vi "4Pi Capture Manager.vi"(7 "Calling VI Ref":refnum<vi>) -> ()   [LabVIEW 2016]
uses:
  4Pi Capture Manager Controls/4Pi Capture Switch Laser.ctl
  4Pi Capture Manager Controls/4Pi Capture Switch Line Scan Modes.ctl
  4Pi Capture Manager Controls/4Pi Capture Line Scan Settings.ctl
  <vilib>/Utility/miscctls.llb/LVPointTypeDef.ctl
  4Pi Capture Manager Controls/4Pi Capture Notifier Type.ctl
  4Pi Capture Manager Controls/4Pi Capture Actions.ctl
  <vilib>/vision/Image Controls.llb/IMAQ Image.ctl
  Hardware Configuration/Hardware Configuration Controls/Device Type.ctl
  Hardware Configuration/Hardware Configuration Controls/Device Function.ctl
  Device Library/Cameras/Hamamatsu/Orca Flash/Orca Flash Controls/Orca Flash Actions.ctl
  Device Library/Cameras/Hamamatsu/Orca Flash/Orca Flash Controls/Orca Flash Parameters.ctl
  Device Library/Cameras/Hamamatsu/Orca Flash/Orca Flash Controls/Orca Flash Parameter List.ctl
  Device Library/Cameras/Hamamatsu/Orca Flash/Orca Flash Controls/Orca Flash ROI.ctl
  4Pi Capture Manager Controls/4Pi Capture Scan Tracker.ctl
  Device Manager/Common Device Queue/Common Device Controls/Common Device Actions.ctl
  Device Library/DAQmx/AO Single Channel Triggered Ramp/AO SCTR Type Defs/AO SCTR Actions.ctl
  Device Library/Stages/Stages Controls/Stage Actions.ctl
  Device Library/Shutters/Shutter Controls/Shutter Actions.ctl
  Device Library/AOTF and AOM/AOTF Controls/AOTF Actions.ctl
  Device Library/Cameras/Camera Controls/Camera IMAQ Key Info.ctl
  <vilib>/Utility/file.llb/Read Delimited Spreadsheet (DBL).vi
  shell32.dll
panel:
  in  "Main Tab":T1(tab)
  out "Frame":u32(slide) scale=0.0..15.0
  out "Cycle":sgl(slide) scale=0.0..1.0
  in  "Base Save Path":path
  in  "Capture":bool
  in  "Live Preview":bool
  in  "Auto Shutter":bool=TRUE
  out "Z Step":sgl(slide) scale=0.0..1.0
  in  "File Name":string="Test Image"
  in  "Preview Exposure Time (s)":dbl=0.1 caption="Frame Rate (Hz)"
  in  "Capture Exposure Time (s)":dbl=0.1 caption="Frame Rate (Hz)"
  in  "No. of Frames":u32=1 min=1
  in  "No. of Cycles":u16=1 min=1
  in  "No. of Z Steps":u16=1 min=1
  in  "Z Step Size (µm)":dbl min=-10.0 max=10.0
  in  "Switch Laser At":T2=enum."Each Cycle"
  in  "Drift Correction":bool
  out "Current Cycle":u16
  out "Current Step":u16
  out "Current Frame":u32
  in  "Auto Update Subfolder":bool=TRUE
  in  "Subfolder Name":string="Area"
  in  "Current Laser":u16(ring)
  in  "Save As Preset":bool
  in  "Line Scan Active":bool
  in  "Number of Lines":u32=8 min=1 max=200 step=1
  in  "Line Scan Mode":T3
  in  "Line Scanning Presets":u16(ring) items=["01 FPS", "02 FPS", "04 FPS", "08 FPS", "16 FPS", "40 FPS"]
  in  "Line Scan Settings":T4
  in  "Camera Settings":bool
  in  "Quadrants On/Off":bool
  in  "Quit":bool
  # "Live Preview"
  # "Capture"
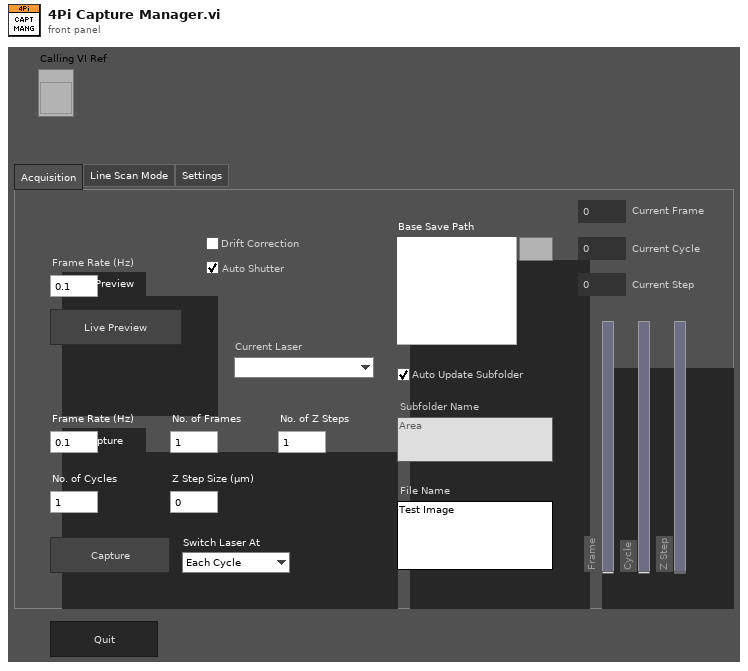
[diagram p1: front panel]
types:
  T1 = enum32{"Acquisition", "Line Scan Mode", "Settings"}
  T2 = typedef "4Pi Capture Switch Laser.ctl" = enum16{"Each Step", "Each Cycle", "All Cycles"}
  T3 = typedef "4Pi Capture Switch Line Scan Modes.ctl" = enum32{"Automatic", "Use Presets", "Manual"}
  T4 = typedef "4Pi Capture Line Scan Settings.ctl" = cluster{"Interline Interval":dbl, "Offset (V)":dbl, "Amplitude (V)":dbl, "Samples Per Channel":dbl, "Delay (ms)":dbl}
  T5 = enum8{"Enabled", "Disabled", "Disabled and Grayed Out"}
  T6 = typedef "Device Type.ctl" = enum16{"AOTF", "Camera", "Deformable Mirror", "Laser", "Shutter", "Stage", "Waveform"}
  T7 = typedef "IMAQ Image.ctl" = refnum<image>
  T8 = typedef "4Pi Capture Notifier Type.ctl" = cluster{"Actions":T9, "Running?":bool, "Preview Exposure (s)":dbl, "Capture Exposure (s)":dbl, "Cycles":u16, "Frames":u32, "No. of Z Steps":u16, "Z Step Size (µm)":dbl, "Base Path":path, "Init Z Position (µm)":dbl, "Lasers Lines":string[], "Save Path":path, "Line Scan?":bool, "Line Scan Mode":T3}
  T9 = typedef "4Pi Capture Actions.ctl" = enum16{"Idle", "Live Preview", "Capture", "Laser On", "Laser Off", "Open Shutters", "Close Shutters", "Set Exposure Time", "Start Acquisition", "Update SubFolder", "Setup", "Camera", "Switch", "Step", "Cycle", "Drift Correction", "Abort", "Quit"}
  T10 = enum16{"Always On", "Always Off", "Off While Running"}
  T11 = typedef "LVPointTypeDef.ctl" = cluster{"Horizontal":i16, "Vertical":i16}
  T12 = typedef "Image Type" = u32
  T13 = typedef "Device Function.ctl" = enum16{"Primary", "Secondary", "Overview", "Wide Field Drift Correction", "642 nm Excitation", "560 nm Excitation", "546 nm Excitation", "488 nm Excitation", "405 nm Excitation", "Objective Drift Correction", "Objective XY", "Objective Z", "Sample XY", "Sample Coarse Z", "Sample Z", "4Pi Lower", "4Pi Upper", "Adj Cavity", "Line Scanning"}
  T14 = typedef "Orca Flash ROI.ctl" = cluster{"H Offset":i32, "V Offset":i32, "H Width":i32, "V Width":i32}
  T15 = typedef "Orca Flash Parameters.ctl" = cluster{"Value":dbl, "Parameter":T16}
  T16 = typedef "Orca Flash Parameter List.ctl" = u32
  T17 = typedef "Orca Flash Actions.ctl" = enum16{"IDLE", "PREVIEW", "RECORD", "Record Settings", "SETPARAM", "GETPARAM", "SETROI", "GETROI", "PROGRESSIVE MODE", "AREA MODE", "STATUS", "QUIT"}
  T18 = typedef "4Pi Capture Scan Tracker.ctl" = cluster{"Current Step":u16, "Current Cycle":u16, "Current Laser":u16, "# of Lasers":u16, "# of Cycles":u16, "# of Steps":u16, "Switch Laser At":T2}
  T19 = typedef "Stage Actions.ctl" = enum16{"Get Position", "MVR", "MOVE", "HALT", "ONTARGET", "ERROR", "REFERENCE", "INIT", "VELOCITY", "STATUS", "EXIT", "HOME", "ZEROPOS", "NANOPOS", "ANALOG", "QUIT"}
  T20 = typedef "Shutter Actions.ctl" = enum16{"Open", "Close", "Toggle", "Status", "Quit"}
  T21 = typedef "AOTF Actions.ctl" = enum16{"Error Check", "Blank", "Line On/Off", "Set Power", "Status", "Quit"}
  T22 = typedef "AO SCTR Actions.ctl" = enum16{"Stop at Offset", "Update and Run", "Quit"}
  T23 = typedef "Camera IMAQ Key Info.ctl" = cluster{"Frame":u32, "Sensor Height":i32, "Sensor Width":i32, "ROI Height":i32, "ROI Width":i32, "ROI Enable?":bool, "Bit per Pixel":u8}
  T24 = typedef "Common Device Actions.ctl" = enum16{"Open Front Panel", "Close Front Panel", "Quit", "Quit All"}
  T25 = typedef "LVRectTypeDef.ctl" = cluster{"Left":i16, "Top":i16, "Right":i16, "Bottom":i16}
  T26 = typedef "LVBoundsTypeDef.ctl" = cluster{"Width":u32, "Height":u32}
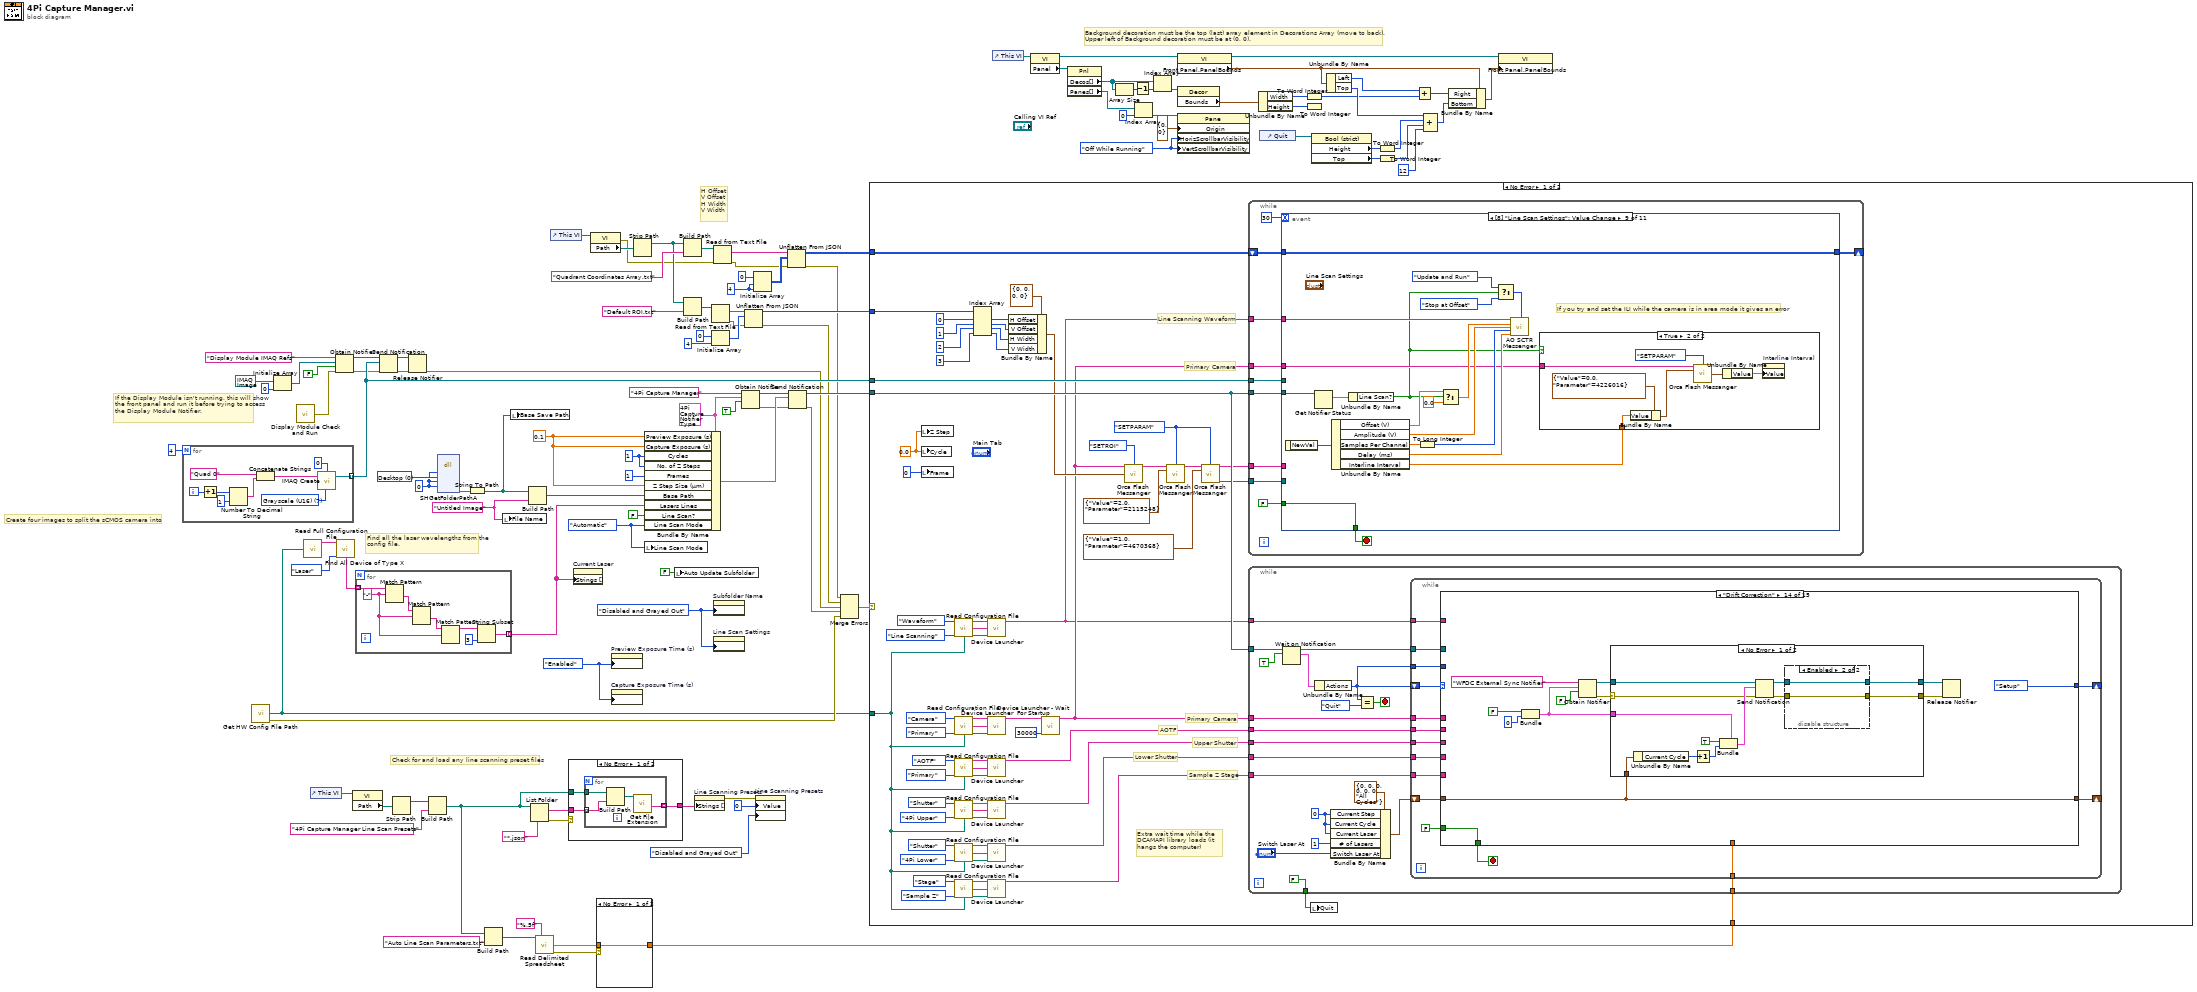
[diagram p0: block diagram]
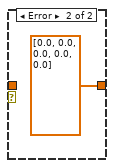
[diagram p2: hidden frame]
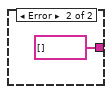
[diagram p3: hidden frame]
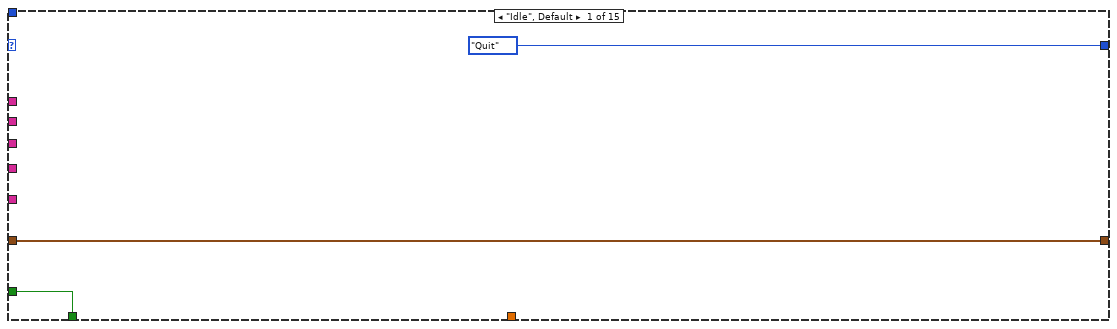
[diagram p4: hidden frame]
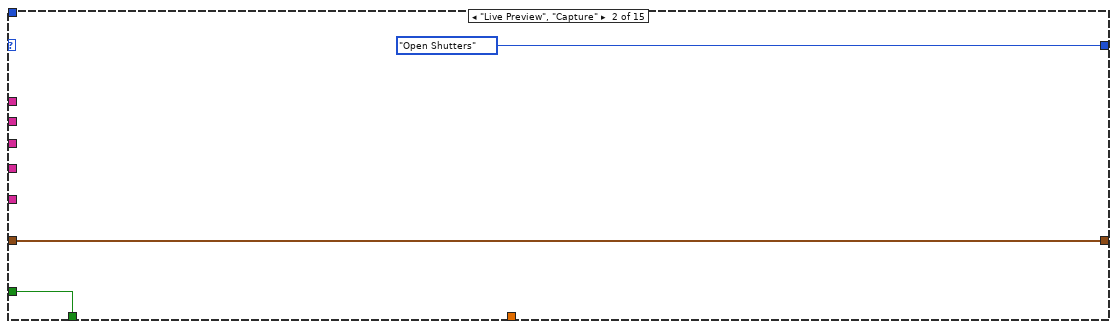
[diagram p5: hidden frame]
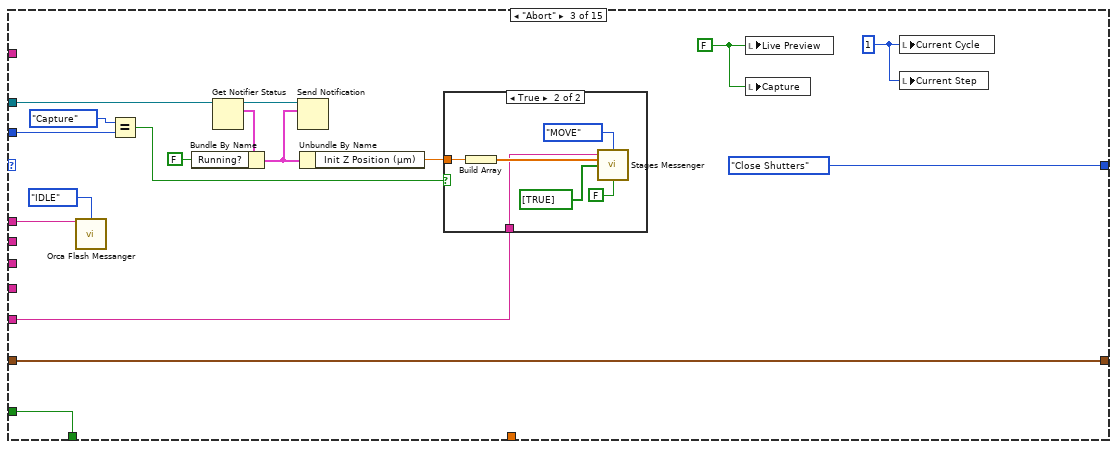
[diagram p6: hidden frame]
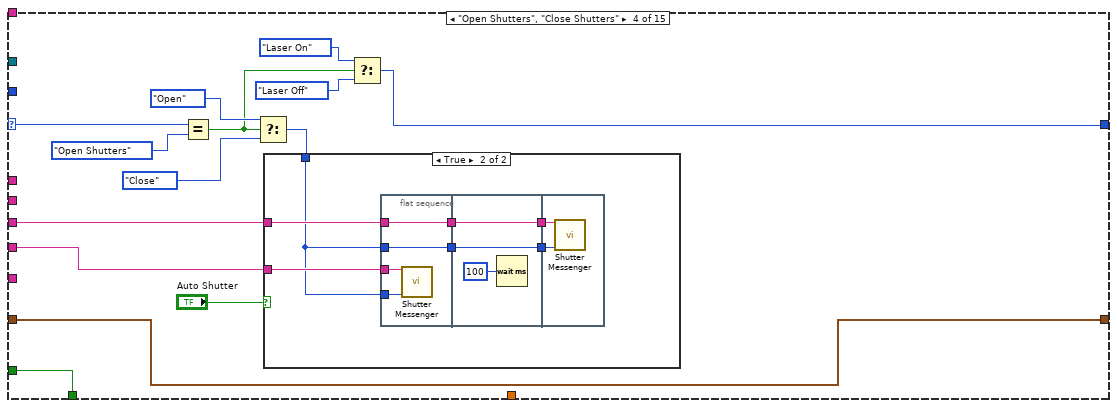
[diagram p8: hidden frame]
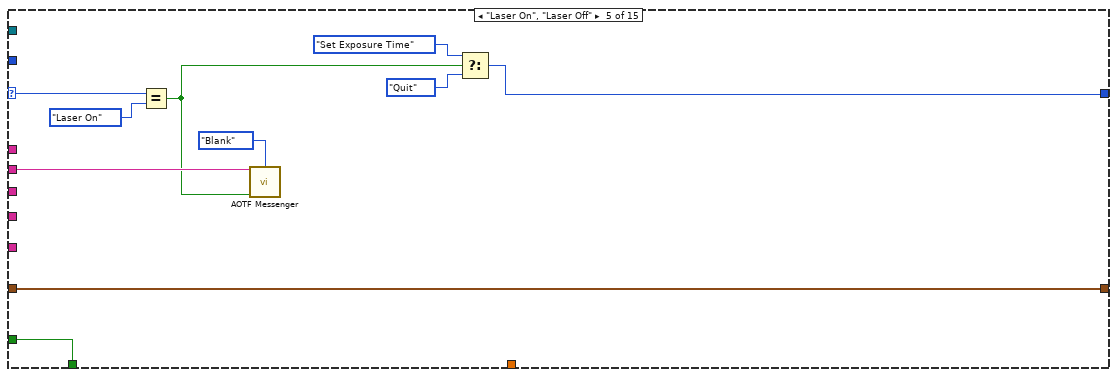
[diagram p10: hidden frame]
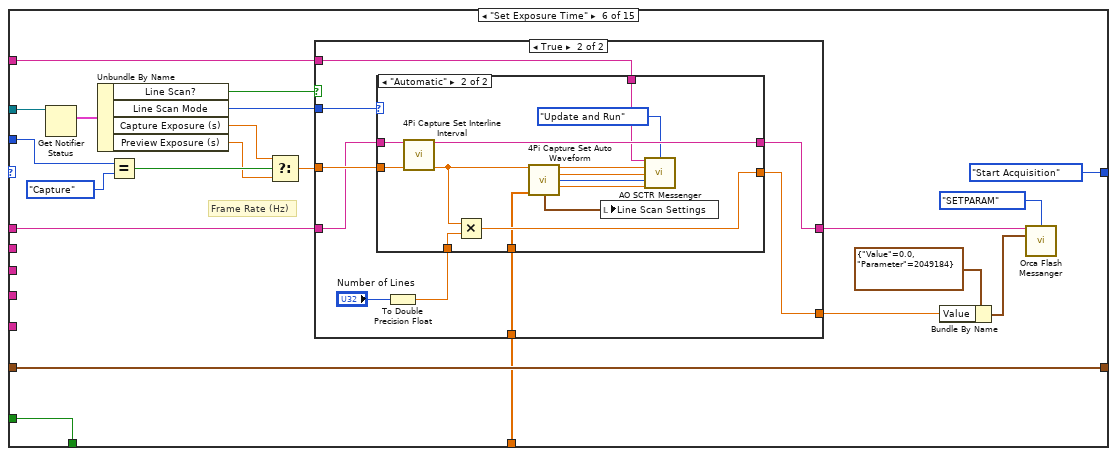
[diagram p11: hidden frame]
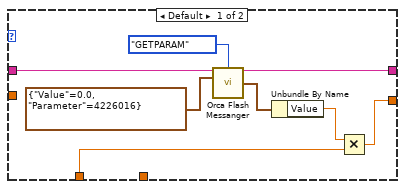
[diagram p13: hidden frame]
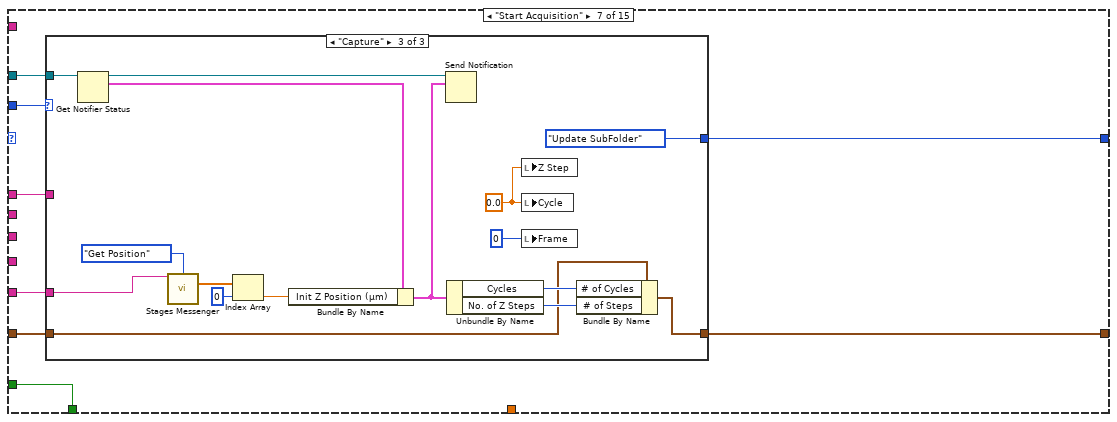
[diagram p14: hidden frame]
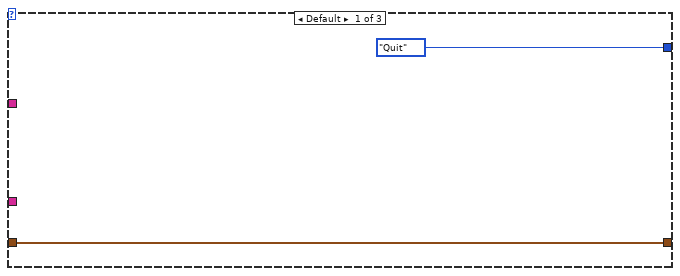
[diagram p15: hidden frame]
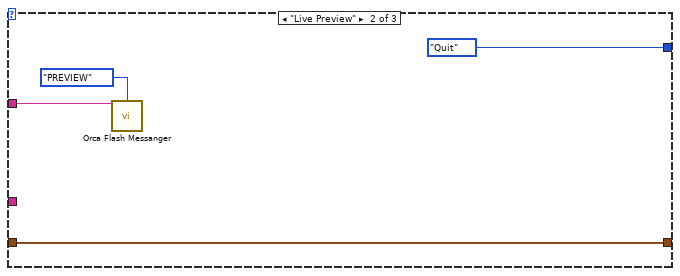
[diagram p16: hidden frame]
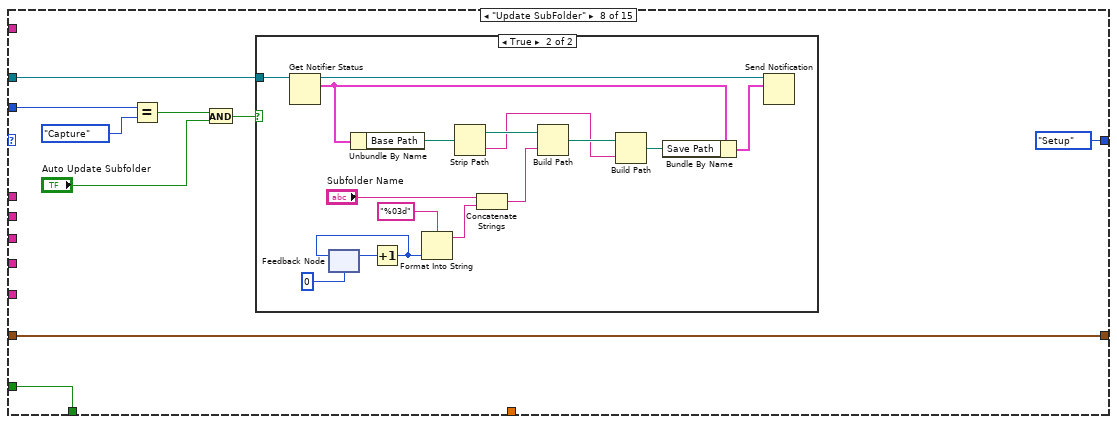
[diagram p17: hidden frame]
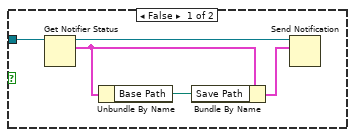
[diagram p18: hidden frame]
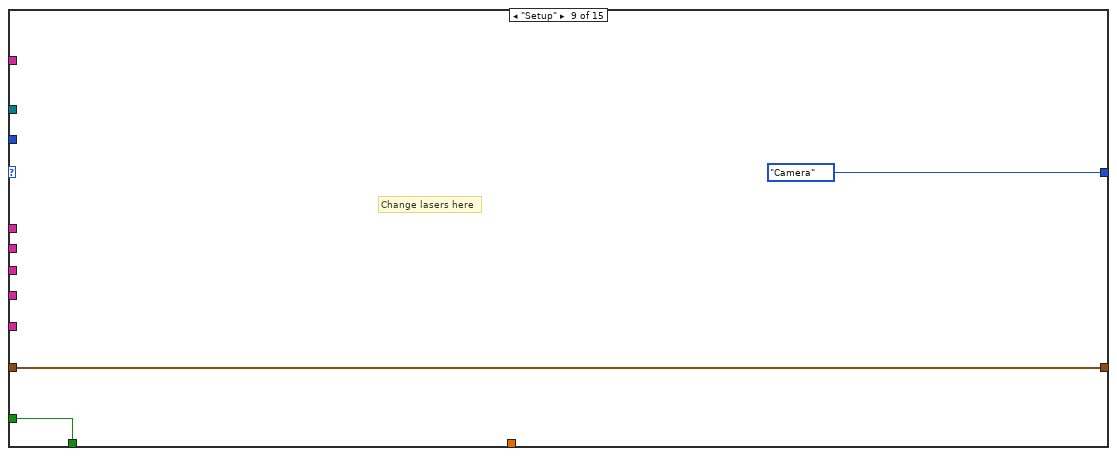
[diagram p19: hidden frame]
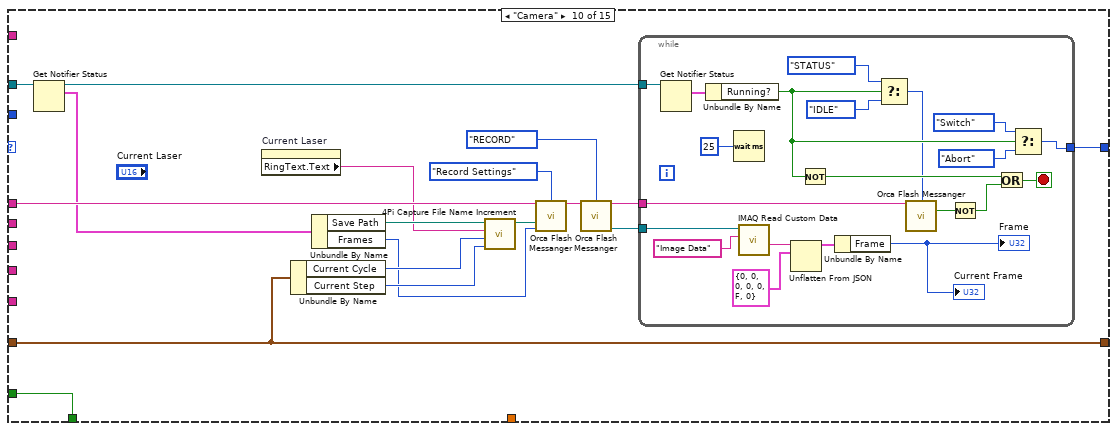
[diagram p20: hidden frame]
diagram:
  w9 = T5."Enabled" ("Disabled")
  w10 = 4Pi_Capture_Switch_Line_Scan_Modes."Automatic" ("Line Scan Mode")
  w11 = T5."Disabled and Grayed Out" ("Disabled")
  w59 = 4 ("dimension size")
  w63 = "Untitled Image"
  w66 = 0 items=["Desktop"=0, "Personal Documents"=5, "AppData"=26, "Local AppData"=28, "Common AppData"=35, "Program Files"=38, "Program Files Common"=43, "Common Documents"=46] ("Requested Path")
  w65 = 0 ("HWND")
  w70 = u16 1 ("Cycles")
  w68 = 0.1 ("Preview Exposure (s)")
  w72 = T8 {"Actions"=enum."Live Preview", "Running?"=FALSE, "Preview Exposure (s)"=0.1, "Capture Exposure (s)"=0.1, "Cycles"=1, "Frames"=0, "No. of Z Steps"=0, "Z Step Size (µm)"=0.0, "Base Path"=path "", "Init Z Position (µm)"=0.0, "Lasers Lines"=[], "Save Path"=path "", "Line Scan?"=FALSE, "Line Scan Mode"=enum."Automatic"} ("4Pi Capture Notifier Type")
  w94 = T10."Off While Running" ("Vertical Scrollbar Visibility")
  # "Check for and load any line scanning preset files"
  # "Find all the laser wavelengths from the config file."
  # "If the Display Module isn't running, this will show the front panel and run it before trying to access the Display Module Notifier."
  # "H Offset\nV Offset\nH Width\nV Width"
  # "Create four images to split the sCMOS camera into"
  # "Background decoration must be the top (last) array element in Decorations Array (move to back).\nUpper left of Background decoration must be at (0, 0)."
  n1 = for {
    N: 4 -> [_]
    tunnel: [w112] -> w76 mode=indexing
    i -> [w120]
    w115 = T12 7 items=["Grayscale (U8)", "Grayscale (I16)", "Grayscale (SGL)", "Complex (CSG)", "RGB (U32)", "HSL (U32)", "RGB (U64)", "Grayscale (U16)"] ("Image Type")
    n2 = Increment(x=w120) -> (x+1=w118:i32)
    n3 = Number To Decimal String(number=w118, width (-)=i16 1) -> (decimal integer string=w116:string)
    n4 = Concatenate Strings("Quad 0" ("name (unnamed)"), w116) -> (w113:string)
    n5 = call "IMAQ Create"("Border Size"=0, "Image Name"=w113, "Image Type"=w115) -> ("New Image"=w112:T7)  [unwired: 2 in, 1 out]
  }
  n6 = call "Get HW Config File Path.vi"() -> ("File Path"=w25:path, "Error"=w39:errorcluster)  [unwired: 14 in]
  n7 = Initialize Array(T7 refnum ("New Image"), 0 ("dimension size")) -> (w30:T7[])
  n8 = call "Display Module Check and Run.vi"() -> ("Error"=w29:errorcluster)  [unwired: 15 in]
  n9 = call "Read Full Configuration File.vi"("Config File Path"=w25) -> ("Unique Notifier Names"=w26:string[])  [unwired: 11 in, 3 out]
  n10 = control-ref of="This VI"() -> (w22:refnum<vi>)
  n11 = Obtain Notifier(name (unnamed)="Display Module IMAQ Refs", notification data type=w30, create if not found? (T)=FALSE, error in (no error)=w29) -> (notifier out=w77:refnum<notifier>, error out=w41:errorcluster)  [unwired: 1 out]
  n12 = call "Find All Device of Type X.vi"("Unique Notifier Names"=w26, "Device Type"=Device_Type."Laser") -> ("All Devices"=w28:string[])  [unwired: 12 in, 1 out]
  n13 = property class="VI"(reference=w22) -> ("Path"=w21:path)  [unwired: 1 in, 2 out]
  n14 = for {
    tunnel: w28 -> [w122] mode=indexing
    tunnel: [w121] -> w1 mode=indexing
    w125 = "-" ("regular expression")
    n15 = Match Pattern(string=w122, regular expression=w125) -> (after substring=w123:string)  [unwired: 1 in, 3 out]
    n16 = Match Pattern(string=w123, regular expression=w125) -> (after substring=w124:string)  [unwired: 1 in, 3 out]
    n17 = Match Pattern(string=w124, regular expression=w125) -> (before substring=w126:string)  [unwired: 1 in, 3 out]
    n18 = String Subset(string=w126, length (rest)=3 ("length (rest)")) -> (substring=w121:string)  [unwired: 1 in]
  }
  n19 = Send Notification(notification=w76, notifier=w77, error in (no error)=w41) -> (notifier out=w61:refnum<notifier>, error out=w46:errorcluster)
  n20 = Strip Path(path=w21) -> (stripped path=w20:path)  [unwired: 1 out]
  n21 = Release Notifier(notifier=w61, error in (no error)=w46) -> (error out=w37:errorcluster)  [unwired: 1 in, 2 out]
  n22 = Build Path(base path=w20, name or relative path="4Pi Capture Manager Line Scan Presets") -> (appended path=w8:path)
  n23 = dll-call lib="shell32.dll" fn="SHGetFolderPathA"("HWND"=w65, "nFolder"=w66, "hToken"=w65, "dwFlags"=w65) -> ("pszPath"=w64:string)  [unwired: 9 in, 2 out]
  n24 = String To Path(string=w64) -> (path=w62:path)
  n25 = Build Path(base path=w8, name or relative path="Auto Line Scan Parameters.txt") -> (appended path=w6:path)
  n26 = local write "File Name"(w63) -> ()
  n27 = local write "Base Save Path"(w62) -> ()
  n28 = Build Path(base path=w62, name or relative path=w63) -> (appended path=w67:path)
  n29 = List Folder(path=w8, pattern="*.json") -> (filenames=w17:string[], error out=w16:errorcluster)  [unwired: 2 in, 2 out]
  n30 = call-poly <vilib>:"Read Delimited Spreadsheet.vi"("file path (dialog if empty)"=w6, "format (%.3f)"="%.5f") -> ("first row"=w3:dbl[], "error out"=w4:errorcluster)  [unwired: 8 in, 4 out]
  n31 = control-ref of="This VI"() -> (w75:refnum<vi>)
  n32 = case shown="No Error" w16 {
    tunnel: w17 -> [w130 _]
    tunnel: w8 -> [w129 _]
    tunnel: [w128 string[] []] -> w15
    frame No Error {
      n33 = for {
        tunnel: w130 -> [w133] mode=indexing
        tunnel: w129 -> [w134]
        tunnel: [w131] -> w128 mode=indexing
        n34 = Build Path(base path=w134, name or relative path=w133) -> (appended path=w132:path)
        n35 = call <vilib>:"Get File Extension.vi"("file"=w132) -> ("filename without extension"=w131:string)  [unwired: 6 in, 4 out]
      }
    }
    frame Error {
    }
  }
  n36 = property on="Current Laser" class="Ring (strict)"("Strings []"=w1) -> ()  [unwired: 2 in, 2 out]
  n37 = property class="VI"(reference=w75) -> (error out=w43:errorcluster, "Path"=w74:path)  [unwired: 1 in, 1 out]
  n38 = case shown="No Error" w4 {
    tunnel: w3 -> [w136 _]
    tunnel: [w136 dbl[] [0.0, 0.0, 0.0, 0.0, 0.0] ("first row")] -> w2
    frame No Error {
    }
    frame Error {
    }
  }
  n39 = property on="Preview Exposure Time (s)" class="DigNum (strict)"("DisabledEnum"=w9) -> ()  [unwired: 2 in, 2 out]
  n40 = property on="Capture Exposure Time (s)" class="DigNum (strict)"("DisabledEnum"=w9) -> ()  [unwired: 2 in, 2 out]
  n41 = Strip Path(path=w74) -> (stripped path=w54:path)  [unwired: 1 out]
  n42 = Bundle By Name(cluster=w72, "Preview Exposure (s)"=w68, "Capture Exposure (s)"=w68, "Cycles"=w70, "No. of Z Steps"=w70, "Frames"=u32 1, "Z Step Size (µm)"=w68, "Base Path"=w67, "Lasers Lines"=w1, "Line Scan?"=FALSE, "Line Scan Mode"=w10) -> (w71:T8)
  n43 = local write "Line Scan Mode"(w10) -> ()
  n44 = local write "Auto Update Subfolder"(FALSE ("Auto Update Subfolder")) -> ()
  n45 = Build Path(base path=w54, name or relative path="Quadrant Coordinates Array.txt") -> (appended path=w57:path)
  n46 = Build Path(base path=w54, name or relative path="Default ROI.txt") -> (appended path=w52:path)
  n47 = property on="Line Scanning Presets" class="Ring (strict)"("Strings []"=w15) -> (error out=w14:errorcluster)  [unwired: 2 in, 1 out]
  n48 = Read from Text File(file (use dialog)=w52) -> (text=w51:string, error out=w44:errorcluster)  [unwired: 3 in, 2 out]
  n49 = Initialize Array(0 ("element"), 4 ("dimension size")) -> (w48:i32[])
  n50 = Read from Text File(file (use dialog)=w57, error in=w43) -> (text=w56:string, error out=w42:errorcluster)  [unwired: 2 in, 2 out]
  n51 = property on="Subfolder Name" class="Str"("DisabledEnum"=w11) -> ()  [unwired: 2 in, 2 out]
  n52 = property on="Line Scan Settings" class="Clust (strict)"("DisabledEnum"=w11) -> ()  [unwired: 2 in, 2 out]
  n53 = Obtain Notifier(name (unnamed)="4Pi Capture Manager", notification data type=w72, create if not found? (T)=TRUE) -> (notifier out=w80:refnum<notifier>, error out=w45:errorcluster)  [unwired: 1 in, 1 out]
  n54 = Unflatten From JSON(JSON string=w51, type and defaults=w48, error in (no error)=w44) -> (value=w47:i32[], error out=w36:errorcluster)  [unwired: 4 in]
  n55 = Initialize Array(0 ("element"), w59, w59) -> (w58:i32[][])
  n56 = property on="Line Scanning Presets" class="Ring (strict)"(error in=w14, "Value"=u16 0, "DisabledEnum"=T5."Disabled and Grayed Out" ("Disabled")) -> ()  [unwired: 1 in, 2 out]
  n57 = Unflatten From JSON(JSON string=w56, type and defaults=w58, error in (no error)=w42) -> (value=w55:i32[][], error out=w35:errorcluster)  [unwired: 4 in]
  n58 = Send Notification(notification=w71, notifier=w80, error in (no error)=w45) -> (notifier out=w79:refnum<notifier>, error out=w38:errorcluster)
  n59 = Merge Errors(w35, w36, w37, w38, w39) -> (w40:errorcluster)
  n60 = case shown="No Error" w40 {
    tunnel: w25 -> [w141 _]
    tunnel: w79 -> [w182 w903]
    tunnel: w76 -> [w168 w901]
    tunnel: w55 -> [w167 _]
    tunnel: w47 -> [w158 _]
    tunnel: w2 -> [w138 _]
    frame No Error {
      w163 = Orca_Flash_Actions."SETPARAM" ("Camera Actions")
      w176 = sgl 0.0 ("Cycle")
      # "Line Scanning Waveform"
      # "Primary Camera"
      # "Extra wait time while the DCAMAPI library loads (it hangs the computer)"
      # "Sample Z Stage"
      # "Lower Shutter"
      # "Upper Shutter"
      # "AOTF"
      # "Primary Camera"
      n61 = local write "Z Step"(w176) -> ()
      n62 = local write "Cycle"(w176) -> ()
      n63 = local write "Frame"(u32 0 ("Frame")) -> ()
      n64 = call "Read Configuration File.vi"("Device Type"=Device_Type."Waveform", "Device Function"=Device_Function."Line Scanning", "Config File Path"=w141) -> ("Unique Notifier Name"=w143:string, "Device Ports/IDs/Channels"=w144:string[], "Device Engine Path"=w140:path)  [unwired: 9 in, 1 out]
      n65 = call "Read Configuration File.vi"("Device Type"=Device_Type."Camera", "Device Function"=Device_Function."Primary", "Config File Path"=w141) -> ("Unique Notifier Name"=w202:string, "Device Ports/IDs/Channels"=w201:string[], "Device Engine Path"=w200:path)  [unwired: 9 in, 1 out]
      n66 = call "Read Configuration File.vi"("Device Type"=Device_Type."AOTF", "Device Function"=Device_Function."Primary", "Config File Path"=w141) -> ("Unique Notifier Name"=w193:string, "Device Ports/IDs/Channels"=w194:string[], "Device Engine Path"=w195:path)  [unwired: 9 in, 1 out]
      n67 = call "Read Configuration File.vi"("Device Type"=Device_Type."Shutter", "Device Function"=Device_Function."4Pi Upper", "Config File Path"=w141) -> ("Unique Notifier Name"=w183:string, "Device Ports/IDs/Channels"=w192:string[], "Device Engine Path"=w191:path)  [unwired: 9 in, 1 out]
      n68 = call "Read Configuration File.vi"("Device Type"=Device_Type."Shutter", "Device Function"=Device_Function."4Pi Lower", "Config File Path"=w141) -> ("Unique Notifier Name"=w184:string, "Device Ports/IDs/Channels"=w187:string[], "Device Engine Path"=w188:path)  [unwired: 9 in, 1 out]
      n69 = call "Read Configuration File.vi"("Device Type"=Device_Type."Stage", "Device Function"=Device_Function."Sample Z", "Config File Path"=w141) -> ("Unique Notifier Name"=w175:string, "Device Ports/IDs/Channels"=w173:string[], "Device Engine Path"=w172:path)  [unwired: 9 in, 1 out]
      n70 = Index Array(array=w158, index #1=0 ("index"), index #2=1 ("index"), index #3=2 ("index"), index #4=3 ("index")) -> (element #1=w153:i32, element #2=w150:i32, element #3=w151:i32, element #4=w152:i32)
      n71 = call "Device Launcher.vi"("Notifier Name"=w143, "Device Ports/IDs/Channels"=w144, "Device Engine Path"=w140) -> ("Notifier Name"=w139:string)  [unwired: 11 in, 1 out]
      n72 = call "Device Launcher.vi"("Notifier Name"=w202, "Device Ports/IDs/Channels"=w201, "Device Engine Path"=w200) -> ("Notifier Name"=w147:string)  [unwired: 11 in, 1 out]
      n73 = call "Device Launcher.vi"("Notifier Name"=w193, "Device Ports/IDs/Channels"=w194, "Device Engine Path"=w195) -> ("Notifier Name"=w181:string)  [unwired: 11 in, 1 out]
      n74 = call "Device Launcher.vi"("Notifier Name"=w183, "Device Ports/IDs/Channels"=w192, "Device Engine Path"=w191) -> ("Notifier Name"=w180:string)  [unwired: 11 in, 1 out]
      n75 = call "Device Launcher.vi"("Notifier Name"=w184, "Device Ports/IDs/Channels"=w187, "Device Engine Path"=w188) -> ("Notifier Name"=w179:string)  [unwired: 11 in, 1 out]
      n76 = call "Device Launcher.vi"("Notifier Name"=w175, "Device Ports/IDs/Channels"=w173, "Device Engine Path"=w172) -> ("Notifier Name"=w170:string)  [unwired: 11 in, 1 out]
      n77 = Bundle By Name(cluster=T14 {"H Offset"=0, "V Offset"=0, "H Width"=0, "V Width"=0} ("Orca Flash ROI"), "H Offset"=w153, "V Offset"=w150, "H Width"=w151, "V Width"=w152) -> (w149:T14)
      n78 = call "Device Launcher - Wait For Startup.vi"("Notifier Name"=w147, "Wait Time (ms)"=30000) -> ("Notifier Name (Dup)"=w146:string)  [unwired: 12 in, 1 out]
      n79 = call "Orca Flash Messanger.vi"("Notifier Name"=w146, "Camera Actions"=Orca_Flash_Actions."SETROI", "sCMOS ROI"=w149) -> ("Notifier Name Dup"=w166:string)  [unwired: 8 in, 4 out]
      n80 = call "Orca Flash Messanger.vi"("Notifier Name"=w166, "Camera Actions"=w163, "sCMOS Parameter"=T15 {"Value"=2.0, "Parameter"=2115248}) -> ("Notifier Name Dup"=w165:string)  [unwired: 8 in, 4 out]
      n81 = call "Orca Flash Messanger.vi"("Notifier Name"=w165, "Camera Actions"=w163, "sCMOS Parameter"=T15 {"Value"=1.0, "Parameter"=4670368}) -> ("Notifier Name Dup"=w164:string, "Image Ref"=w160:T7)  [unwired: 8 in, 3 out]
      n82 = while {
        tunnel: w182 -> [w588]
        tunnel: w164 -> [w587]
        tunnel: w160 -> [w585]
        tunnel: w168 -> [w584]
        shift-right: [w582] -> _
        shift-left: w167 -> [w583]
        tunnel: w146 -> [w581]
        tunnel: w139 -> [w580]
        stop <- w590 stop-if-true
        n83 = event shown="[8] \"Line Scan Settings\": Value Change" {
          selector: _ -> [_ _ _ _ _ _ _ _ _ _ _]
          dyn-events: _ -> [_ _ _ _ _ _ _ _ _ _ _]
          timeout: 30 -> [_ _ _ _ _ _ _ _ _ _ _]
          tunnel: [w595 w613 w686 w707 w763 w788 w810 w826 w846 w870 w899] -> w590
          tunnel: FALSE -> [w595 w613 w686 w707 w763 w788 w810 w826 w846 w870 _]
          tunnel: w588 -> [_ w610 w683 _ _ w782 w808 _ w844 _ w898]
          tunnel: w587 -> [_ w609 _ _ _ _ _ _ _ _ _]
          tunnel: w585 -> [w593 _ _ w691 _ _ _ _ _ _ _]
          tunnel: w584 -> [w594 _ _ w697 _ _ _ _ _ _ w886]
          tunnel: w583 -> [w592 w608 w675 w690 w758 w765 w809 w827 w845 w862 w885]
          tunnel: [w592 w608 w675 w689 w758 w765 w809 w827 w845 w862 w885] -> w582
          tunnel: w581 -> [_ _ _ _ _ w776 _ _ w830 _ _]
          tunnel: w580 -> [_ _ _ _ _ w766 _ _ w838 _ _]
          event Timeout {
            # "Convert to array and then crop. If you\nextract or mask image the destination\nimage custom data keys are overwritten."
            n84 = event-data() -> ()  [unwired: 1 in, 1 out]
            n85 = call "IMAQ ImageToArray"("Image"=w593) -> ("Image Pixels (U16)"=w591:u16[][])  [unwired: 3 in, 4 out]
            n86 = for {
              tunnel: w594 -> [w606] mode=indexing
              tunnel: w591 -> [w607]
              tunnel: w592 -> [w604] mode=indexing
              n87 = Index Array(array=w604, index #1=0 ("index"), index #2=2 ("index"), index #3=1 ("index"), index #4=3 ("index")) -> (element #1=w602:i32, element #2=w601:i32, element #3=w597:i32, element #4=w596:i32)
              n88 = Array Subset(array=w607, index (row)=w602, length (row)=w601, index (col)=w597, length (col)=w596) -> (w605:u16[][])
              n89 = call "IMAQ ArrayToImage"("Image Pixels (U16)"=w605, "Image"=w606) -> ()  [unwired: 8 in, 2 out]
            }
          }
          event "Camera Settings", "Preview Exposure Time (s)", "Capture Exposure Time (s)", "No. of Cycles", "No. of Frames", "No. of Z Steps", "Z Step Size (µm)", "Base Save Path", "File Name": Value Change {
            n90 = event-data() -> ("CtlRef"=w612:refnum<vi>)  [unwired: 1 in]
            n91 = property class="Ctl"(reference=w612) -> ("Label.Text"=w611:string)  [unwired: 1 in, 2 out]
            n92 = case shown="\"Preview Exposure Time (s)\"" w611 {
              tunnel: w610 -> [_ w617 w625 w631 w637 w649 _ w665 w674]
              tunnel: w609 -> [_ _ _ _ _ _ w657 _ _]
              frame Default {
              }
              frame "No. of Cycles" {
                n93 = Get Notifier Status(notifier=w617) -> (notifier out=w616:refnum<notifier>, current notification=w618:T8)  [unwired: 1 in, 3 out]
                n94 = Bundle By Name(cluster=w618, "Cycles"="No. of Cycles", "Actions"=4Pi_Capture_Actions."Idle") -> (w619:T8)
                n95 = Send Notification(notification=w619, notifier=w616) -> ()  [unwired: 1 in, 2 out]
              }
              frame "No. of Frames" {
                n96 = To Double Precision Float(number="No. of Frames") -> (double precision float=w621:dbl)
                n97 = property on="Frame" class="Slide (strict)"("Scale.Maximum"=w621, "Scale.Minimum"=0.0 ("Scale.Range:Minimum")) -> ()  [unwired: 2 in, 2 out]
                n98 = Get Notifier Status(notifier=w625) -> (notifier out=w624:refnum<notifier>, current notification=w626:T8)  [unwired: 1 in, 3 out]
                n99 = Bundle By Name(cluster=w626, "Frames"="No. of Frames", "Actions"=4Pi_Capture_Actions."Idle") -> (w627:T8)
                n100 = Send Notification(notification=w627, notifier=w624) -> ()  [unwired: 1 in, 2 out]
              }
              frame "No. of Z Steps" {
                n101 = Get Notifier Status(notifier=w631) -> (notifier out=w630:refnum<notifier>, current notification=w632:T8)  [unwired: 1 in, 3 out]
                n102 = Bundle By Name(cluster=w632, "No. of Z Steps"="No. of Z Steps", "Actions"=4Pi_Capture_Actions."Idle") -> (w633:T8)
                n103 = Send Notification(notification=w633, notifier=w630) -> ()  [unwired: 1 in, 2 out]
              }
              frame "Z Step Size (µm)" {
                n104 = Get Notifier Status(notifier=w637) -> (notifier out=w636:refnum<notifier>, current notification=w638:T8)  [unwired: 1 in, 3 out]
                n105 = Bundle By Name(cluster=w638, "Z Step Size (µm)"="Z Step Size (µm)", "Actions"=4Pi_Capture_Actions."Idle") -> (w639:T8)
                n106 = Send Notification(notification=w639, notifier=w636) -> ()  [unwired: 1 in, 2 out]
              }
              frame "File Name", "Save Path" {
                n107 = Path To String(path="Base Save Path") -> (string=w644:string)
                n108 = Equal?(x="", y=w644) -> (x = y?=w642:bool)
                n109 = case shown="True" w642 {
                  tunnel: [w652 w653] -> w641
                  tunnel: "Base Save Path" -> [w652 _]
                  frame False {
                  }
                  frame True {
                    w656 = 0 items=["Desktop"=0, "Personal Documents"=5, "AppData"=26, "Local AppData"=28, "Common AppData"=35, "Program Files"=38, "Program Files Common"=43, "Common Documents"=46] ("Requested Path")
                    w655 = 0 ("HWND")
                    n110 = dll-call lib="shell32.dll" fn="SHGetFolderPathA"("HWND"=w655, "nFolder"=w656, "hToken"=w655, "dwFlags"=w655) -> ("pszPath"=w654:string)  [unwired: 9 in, 2 out]
                    n111 = String To Path(string=w654) -> (path=w653:path)
                  }
                }
                n112 = Build Path(base path=w641, name or relative path="File Name") -> (appended path=w645:path)
                n113 = Get Notifier Status(notifier=w649) -> (notifier out=w648:refnum<notifier>, current notification=w650:T8)  [unwired: 1 in, 3 out]
                n114 = Bundle By Name(cluster=w650, "Base Path"=w645, "Actions"=4Pi_Capture_Actions."Idle") -> (w651:T8)
                n115 = Send Notification(notification=w651, notifier=w648) -> ()  [unwired: 1 in, 2 out]
              }
              frame "Camera Settings" {
                n116 = Select(t=Common_Device_Actions."Open Front Panel" ("Common Actions"), s="Camera Settings", f=Common_Device_Actions."Close Front Panel" ("Common Actions")) -> (s? t:f=w661:T24)
                n117 = call "Common Device Queue Messenger.vi"("Common Action"=w661, "Notifier Name"=w657) -> ()  [unwired: 13 in, 1 out]
              }
              frame "Preview Exposure Time (s)" {
                # "Add in a preview stop\nand restart here"
                n118 = Get Notifier Status(notifier=w665) -> (notifier out=w668:refnum<notifier>, current notification=w667:T8)  [unwired: 1 in, 3 out]
                n119 = Bundle By Name(cluster=w667, "Preview Exposure (s)"="Preview Exposure Time (s)", "Running?"=FALSE ("Abort"), "Actions"=4Pi_Capture_Actions."Idle") -> (w666:T8)
                n120 = Send Notification(notification=w666, notifier=w668) -> ()  [unwired: 1 in, 2 out]
              }
              frame "Capture Exposure Time (s)" {
                n121 = Get Notifier Status(notifier=w674) -> (notifier out=w673:refnum<notifier>, current notification=w672:T8)  [unwired: 1 in, 3 out]
                n122 = Bundle By Name(cluster=w672, "Capture Exposure (s)"="Capture Exposure Time (s)", "Actions"=4Pi_Capture_Actions."Idle") -> (w671:T8)
                n123 = Send Notification(notification=w671, notifier=w673) -> ()  [unwired: 1 in, 2 out]
              }
            }
          }
          event "Live Preview", "Capture": Value Change {
            n124 = event-data() -> ("CtlRef"=w678:refnum<vi>, "NewVal"=w681:bool)  [unwired: 1 in]
            n125 = property class="Bool (strict)"(reference=w678) -> ("Label.Text"=w677:string)  [unwired: 1 in, 2 out]
            n126 = case shown="\"Live Preview\", Default" w677 {
              tunnel: [4Pi_Capture_Actions."Capture" ("y") 4Pi_Capture_Actions."Live Preview" ("y")] -> w676
              frame "Capture" {
              }
              frame "Live Preview", Default {
              }
            }
            n127 = Select(t=w676, s=w681, f=4Pi_Capture_Actions."Abort" ("y")) -> (s? t:f=w680:T9)
            n128 = Get Notifier Status(notifier=w683) -> (notifier out=w684:refnum<notifier>, current notification=w682:T8)  [unwired: 1 in, 3 out]
            n129 = Bundle By Name(cluster=w682, "Actions"=w680, "Running?"=w681) -> (w679:T8)
            n130 = Send Notification(notification=w679, notifier=w684) -> ()  [unwired: 1 in, 2 out]
          }
          event "Quadrants On/Off": Value Change {
            n131 = event-data() -> ("NewVal"=w703:bool)  [unwired: 1 in]
            n132 = Obtain Notifier(name (unnamed)="Display Module IMAQ Refs", notification data type=T7[] [], create if not found? (T)=FALSE) -> (notifier out=w696:refnum<notifier>, error out=w695:errorcluster)  [unwired: 1 in, 1 out]
            n133 = Get Notifier Status(notifier=w696, error in (no error)=w695) -> (notifier out=w694:refnum<notifier>, current notification=w692:T7[], error out=w693:errorcluster)  [unwired: 2 out]
            n134 = case shown="False" w703 {
              tunnel: w694 -> [w729 w744]
              tunnel: w693 -> [w728 w743]
              tunnel: [w725 w739] -> w699
              tunnel: [w729 w744] -> w700
              tunnel: [w728 w743] -> w698
              tunnel: w697 -> [w720 w742]
              tunnel: w692 -> [w727 w741]
              tunnel: w691 -> [w721 w738]
              tunnel: w690 -> [_ w737]
              tunnel: [w708 w737] -> w689
              frame False {
                w719 = 4 ("dimension size")
                n135 = control-ref of="This VI"() -> (w709:refnum<vi>)
                n136 = Equal?(x=w727, y=w721) -> (x = y?=w724:bool[])
                n137 = property class="VI"(reference=w709) -> (error out=w717:errorcluster, "Path"=w710:path)  [unwired: 1 in, 1 out]
                n138 = for {
                  tunnel: w724 -> [w736] mode=indexing
                  tunnel: [w735] -> w722
                  i -> [w735]
                  stop <- w736 stop-if-true
                }
                n139 = Or Array Elements(Boolean array=w724) -> (logical OR=w723:bool)
                n140 = Strip Path(path=w710) -> (stripped path=w716:path)  [unwired: 1 out]
                n141 = case shown="True" w723 {
                  tunnel: w722 -> [_ w733]
                  tunnel: w727 -> [w730 w732]
                  tunnel: [w730 w731] -> w726
                  frame False {
                  }
                  frame True {
                    n142 = Delete From Array(array=w732, length=1, index=w733) -> (array with subset deleted=w731:T7[])  [unwired: 1 out]
                  }
                }
                n143 = Build Path(base path=w716, name or relative path="Quadrant Coordinates Array.txt") -> (appended path=w714:path)
                n144 = Read from Text File(file (use dialog)=w714, error in=w717) -> (text=w715:string, error out=w718:errorcluster)  [unwired: 2 in, 2 out]
                n145 = Initialize Array(0 ("element"), w719, w719) -> (w713:i32[][])
                n146 = Build Array (concatenate)(w726, w720) -> (w725:T7[])
                n147 = Unflatten From JSON(JSON string=w715, type and defaults=w713, error in (no error)=w718) -> (value=w708:i32[][])  [unwired: 4 in, 1 out]
              }
              frame True {
                n148 = for {
                  tunnel: w742 -> [w747] mode=indexing
                  shift-right: [w745] -> w740
                  shift-left: w741 -> [w746]
                  n149 = Equal?(x=w746, y=w747) -> (x = y?=w750:bool[])
                  n150 = for {
                    tunnel: w750 -> [w757] mode=indexing
                    tunnel: [w756] -> w748
                    i -> [w756]
                    stop <- w757 stop-if-true
                  }
                  n151 = Or Array Elements(Boolean array=w750) -> (logical OR=w749:bool)
                  n152 = case shown="True" w749 {
                    tunnel: w748 -> [_ w754]
                    tunnel: w746 -> [w751 w753]
                    tunnel: [w751 w752] -> w745
                    frame False {
                    }
                    frame True {
                      n153 = Delete From Array(array=w753, length=1, index=w754) -> (array with subset deleted=w752:T7[])  [unwired: 1 out]
                    }
                  }
                }
                n154 = Build Array (concatenate)(w740, w738) -> (w739:T7[])
              }
            }
            n155 = Send Notification(notification=w699, notifier=w700, error in (no error)=w698) -> (notifier out=w702:refnum<notifier>, error out=w701:errorcluster)
            n156 = Release Notifier(notifier=w702, error in (no error)=w701) -> ()  [unwired: 1 in, 3 out]
          }
          event "Auto Update Subfolder": Value Change {
            n157 = event-data() -> ("NewVal"=w762:bool)  [unwired: 1 in]
            n158 = Select(t=T5."Enabled" ("Disabled"), s=w762, f=T5."Disabled and Grayed Out") -> (s? t:f=w759:T5)
            n159 = property on="Subfolder Name" class="Str"("DisabledEnum"=w759) -> ()  [unwired: 2 in, 2 out]
          }
          event "Line Scan Active": Value Change {
            n160 = event-data() -> ("NewVal"=w764:bool)  [unwired: 1 in]
            n161 = Select(t="Frame Rate (Hz)", s=w764, f="Exposure Time (s)") -> (s? t:f=w785:string)
            n162 = Select(t=4.0, s=w764, f=0.1) -> (s? t:f=w778:dbl)
            n163 = Select(t=-1.0 ("f"), s=w764, f=0.0) -> (s? t:f=w769:dbl)
            n164 = Select(t=AO_SCTR_Actions."Update and Run" ("Actions"), s=w764, f=AO_SCTR_Actions."Stop at Offset" ("Actions")) -> (s? t:f=w770:T22)
            n165 = property on="Capture Exposure Time (s)" class="DigNum (strict)"("Caption.Text"=w785, "Value"=w778) -> ()  [unwired: 2 in, 2 out]
            n166 = property on="Preview Exposure Time (s)" class="DigNum (strict)"("Caption.Text"=w785, "Value"=w778) -> ()  [unwired: 2 in, 2 out]
            n167 = call "AO SCTR Messenger.vi"("Notifier Name"=w766, "Actions"=w770, "Offset (V)"=w769) -> ()  [unwired: 12 in, 1 out]
            n168 = case shown="False" w764 {
              frame False {
                w789 = T5."Enabled" ("Disabled")
                n169 = property on="Preview Exposure Time (s)" class="DigNum (strict)"("DisabledEnum"=w789) -> ()  [unwired: 2 in, 2 out]
                n170 = property on="Capture Exposure Time (s)" class="DigNum (strict)"("DisabledEnum"=w789) -> ()  [unwired: 2 in, 2 out]
              }
              frame True {
              }
            }
            n171 = Get Notifier Status(notifier=w782) -> (notifier out=w781:refnum<notifier>, current notification=w780:T8)  [unwired: 1 in, 3 out]
            n172 = Bundle By Name(cluster=w780, "Line Scan?"=w764, "Actions"=4Pi_Capture_Actions."Idle", "Preview Exposure (s)"=w778, "Capture Exposure (s)"=w778) -> (w777:T8)
            n173 = Select(t=Orca_Flash_Actions."PROGRESSIVE MODE" ("Camera Actions"), s=w764, f=Orca_Flash_Actions."AREA MODE" ("Camera Actions")) -> (s? t:f=w773:T17)
            n174 = call "Orca Flash Messanger.vi"("Notifier Name"=w776, "Camera Actions"=w773) -> ()  [unwired: 9 in, 5 out]
            n175 = Send Notification(notification=w777, notifier=w781) -> ()  [unwired: 1 in, 2 out]
          }
          event Value Change {
            n176 = event-data() -> ("NewVal"=w799:T3)  [unwired: 1 in]
            n177 = Get Notifier Status(notifier=w808) -> (notifier out=w807:refnum<notifier>, current notification=w806:T8)  [unwired: 1 in, 3 out]
            n178 = Bundle By Name(cluster=w806, "Actions"=4Pi_Capture_Actions."Idle", "Line Scan Mode"=w799) -> (w805:T8)
            n179 = Send Notification(notification=w805, notifier=w807) -> ()  [unwired: 1 in, 2 out]
            n180 = Equal?(x=w799, y=4Pi_Capture_Switch_Line_Scan_Modes."Use Presets") -> (x = y?=w791:bool)
            n181 = Not Equal?(x=w799, y=4Pi_Capture_Switch_Line_Scan_Modes."Automatic") -> (x != y?=w793:bool)
            n182 = Select(t=T5."Enabled" ("Disabled"), s=w791, f=T5."Disabled and Grayed Out" ("Disabled")) -> (s? t:f=w801:T5)
            n183 = property on="Line Scanning Presets" class="Ring (strict)"("DisabledEnum"=w801) -> ()  [unwired: 2 in, 2 out]
            n184 = case shown="True" w791 {
              frame False {
              }
              frame True {
                n185 = property on="Line Scanning Presets" class="Ring (strict)"() -> ("Value"=w811:u16)  [unwired: 2 in, 2 out]
                n186 = property on="Line Scanning Presets" class="Ring (strict)"("Val(Sgnl)"=w811) -> ()  [unwired: 2 in, 2 out]
              }
            }
            n187 = Select(t=T5."Disabled and Grayed Out" ("Disabled"), s=w793, f=T5."Enabled" ("Disabled")) -> (s? t:f=w792:T5)
            n188 = Select(t=T5."Enabled" ("Disabled"), s=w793, f=T5."Disabled and Grayed Out" ("Disabled")) -> (s? t:f=w796:T5)
            n189 = property on="Preview Exposure Time (s)" class="DigNum (strict)"("DisabledEnum"=w792) -> ()  [unwired: 2 in, 2 out]
            n190 = property on="Capture Exposure Time (s)" class="DigNum (strict)"("DisabledEnum"=w792) -> ()  [unwired: 2 in, 2 out]
            n191 = property on="Save As Preset" class="Bool"("DisabledEnum"=w796) -> ()  [unwired: 2 in, 2 out]
            n192 = property on="Line Scan Settings" class="Clust (strict)"("DisabledEnum"=w796) -> ()  [unwired: 2 in, 2 out]
          }
          event "Line Scanning Presets": Value Change {
            n193 = event-data() -> ("CtlRef"=w821:refnum<vi>)  [unwired: 1 in]
            n194 = control-ref of="This VI"() -> (w825:refnum<vi>)
            n195 = property class="Ring (strict)"(reference=w821) -> ("RingText.Text"=w819:string)  [unwired: 1 in, 2 out]
            n196 = property class="VI"(reference=w825) -> ("Path"=w824:path)  [unwired: 1 in, 2 out]
            n197 = Strip Path(path=w824) -> (stripped path=w823:path)  [unwired: 1 out]
            n198 = Concatenate Strings(w819, ".json" ("string")) -> (w817:string)
            n199 = Build Path(base path=w823, name or relative path="4Pi Capture Manager Line Scan Presets") -> (appended path=w820:path)
            n200 = Build Path(base path=w820, name or relative path=w817) -> (appended path=w816:path)
            n201 = Read from Text File(file (use dialog)=w816) -> (text=w815:string, error out=w813:errorcluster)  [unwired: 3 in, 2 out]
            n202 = Unflatten From JSON(JSON string=w815, type and defaults=T4 {"Interline Interval"=0.0, "Offset (V)"=0.0, "Amplitude (V)"=0.0, "Samples Per Channel"=0.0, "Delay (ms)"=0.0} ("Line Scan Settings"), error in (no error)=w813) -> (value=w812:T4)  [unwired: 4 in, 1 out]
            n203 = property on="Line Scan Settings" class="Clust (strict)"("Val(Sgnl)"=w812) -> ()  [unwired: 2 in, 2 out]
          }
          event Value Change {
            # "If you try and set the ILI while the camera is in area mode it gives an error"
            n204 = event-data() -> ("NewVal"=w839:T4)  [unwired: 1 in]
            n205 = Get Notifier Status(notifier=w844) -> (current notification=w843:T8)  [unwired: 1 in, 4 out]
            n206 = Unbundle By Name(w839) -> ("Offset (V)"=w833:dbl, "Amplitude (V)"=w837:dbl, "Samples Per Channel"=w836:dbl, "Delay (ms)"=w835:dbl, "Interline Interval"=w829:dbl)
            n207 = Unbundle By Name(w843) -> ("Line Scan?"=w828:bool)
            n208 = To Long Integer(number=w836) -> (32bit integer=w834:i32)
            n209 = Select(t=w833, s=w828, f=0.0) -> (s? t:f=w831:dbl)
            n210 = Select(t=AO_SCTR_Actions."Update and Run" ("Actions"), s=w828, f=AO_SCTR_Actions."Stop at Offset" ("Actions")) -> (s? t:f=w840:T22)
            n211 = call "AO SCTR Messenger.vi"("Notifier Name"=w838, "Actions"=w840, "Offset (V)"=w831, "Amplitude (V)"=w837, "Samples Per Channel"=w834, "Start Delay (ms)"=w835) -> ()  [unwired: 9 in, 1 out]
            n212 = case shown="True" w828 {
              tunnel: w830 -> [_ w849]
              tunnel: w829 -> [_ w848]
              frame False {
              }
              frame True {
                n213 = Bundle By Name(cluster=T15 {"Value"=0.0, "Parameter"=4226016} ("sCMOS Parameter"), "Value"=w848) -> (w852:T15)
                n214 = call "Orca Flash Messanger.vi"("Notifier Name"=w849, "Camera Actions"=Orca_Flash_Actions."SETPARAM", "sCMOS Parameter"=w852) -> ("sCMOS Parameter"=w853:T15)  [unwired: 8 in, 4 out]
                n215 = Unbundle By Name(w853) -> ("Value"=w847:dbl)
                n216 = property on="Interline Interval" class="DigNum (strict)"("Value"=w847) -> ()  [unwired: 2 in, 2 out]
              }
            }
          }
          event "Save As Preset": Value Change {
            n217 = event-data() -> ()  [unwired: 1 in, 6 out]
            n218 = control-ref of="This VI"() -> (w866:refnum<vi>)
            n219 = property class="VI"(reference=w866) -> ("Path"=w865:path)  [unwired: 1 in, 2 out]
            n220 = Strip Path(path=w865) -> (stripped path=w864:path)  [unwired: 1 out]
            n221 = Build Path(base path=w864, name or relative path="4Pi Capture Manager Line Scan Presets") -> (appended path=w855:path)
            n222 = call "File Dialog"("start path"=w855, "prompt"="Save Preset File", "pattern (all files)"="*.json", "pattern label"="JSON") -> ("selected path"=w860:path, "error out"=w861:errorcluster)  [unwired: 8 in, 2 out]
            n223 = case shown="Error" w861 {
              selector: w861 -> [_ w884]
              tunnel: w860 -> [w883 _]
              tunnel: [w879 w884] -> w854
              frame No Error {
                n224 = local read "Line Scan Settings"() -> (w882:T4)
                n225 = Flatten To JSON(anything=w882) -> (JSON string=w881:string, 11:w880:errorcluster)  [unwired: 2 in]
                n226 = Write to Text File(file (use dialog)=w883, text=w881, error in=w880) -> (error out=w879:errorcluster)  [unwired: 1 in, 2 out]
              }
              frame Error {
              }
            }
            n227 = List Folder(path=w855, pattern="*.json", error in=w854) -> (filenames=w858:string[], error out=w857:errorcluster)  [unwired: 1 in, 2 out]
            n228 = case shown="No Error" w857 {
              tunnel: w858 -> [w873 _]
              tunnel: w855 -> [w872 _]
              tunnel: [w871 string[] []] -> w856
              frame No Error {
                n229 = for {
                  tunnel: w873 -> [w876] mode=indexing
                  tunnel: w872 -> [w877]
                  tunnel: [w874] -> w871 mode=indexing
                  n230 = Build Path(base path=w877, name or relative path=w876) -> (appended path=w875:path)
                  n231 = call <vilib>:"Get File Extension.vi"("file"=w875) -> ("filename without extension"=w874:string)  [unwired: 6 in, 4 out]
                }
              }
              frame Error {
              }
            }
            n232 = property on="Line Scanning Presets" class="Ring (strict)"("Strings []"=w856) -> ()  [unwired: 2 in, 2 out]
          }
          event "Quit": Value Change {
            n233 = event-data() -> ("NewVal"=w899:bool)  [unwired: 1 in]
            n234 = Get Notifier Status(notifier=w898) -> (notifier out=w897:refnum<notifier>, current notification=w896:T8)  [unwired: 1 in, 3 out]
            n235 = Bundle By Name(cluster=w896, "Running?"=FALSE ("Abort"), "Actions"=4Pi_Capture_Actions."Quit") -> (w890:T8)
            n236 = Send Notification(notification=w890, notifier=w897) -> (notifier out=w894:refnum<notifier>)  [unwired: 1 in, 1 out]
            n237 = Wait on Notification(notifier=w894, ignore previous (F)=TRUE, timeout in ms (-1)=500) -> (notifier out=w891:refnum<notifier>)  [unwired: 1 in, 3 out]
            n238 = Send Notification(notification=w890, notifier=w891) -> (notifier out=w888:refnum<notifier>)  [unwired: 1 in, 1 out]
            n239 = Release Notifier(notifier=w888, force destroy? (F)=TRUE) -> ()  [unwired: 1 in, 3 out]
            n240 = for {
              tunnel: w886 -> [w900] mode=indexing
              n241 = call "IMAQ Dispose"("Image"=w900) -> ()  [unwired: 5 in, 1 out]
            }
          }
        }
      }
      n242 = while {
        tunnel: w182 -> [w222]
        tunnel: w146 -> [w216]
        tunnel: w181 -> [w214]
        tunnel: w180 -> [w213]
        tunnel: w179 -> [w212]
        tunnel: [FALSE] -> w178
        tunnel: w170 -> [w210]
        tunnel: w139 -> [w204]
        tunnel: w138 -> [w203]
        stop <- w218 stop-if-true
        w208 = u16 0 ("Current Step")
        n243 = Wait on Notification(notifier=w222, ignore previous (F)=TRUE) -> (notifier out=w217:refnum<notifier>, notification=w220:T8)  [unwired: 2 in, 2 out]
        n244 = Unbundle By Name(w220) -> ("Actions"=w215:T9)
        n245 = Bundle By Name(cluster=T18 {"Current Step"=0, "Current Cycle"=0, "Current Laser"=0, "# of Lasers"=0, "# of Cycles"=0, "# of Steps"=0, "Switch Laser At"=enum."All Cycles"} ("Cluster"), "Current Step"=w208, "Current Cycle"=w208, "Current Laser"=w208, "# of Lasers"=u16 1, "Switch Laser At"="Switch Laser At") -> (w206:T18)
        n246 = Equal?(x=w215, y=4Pi_Capture_Actions."Quit") -> (x = y?=w218:bool)
        n247 = while {
          shift-right: [w236] -> _
          shift-left: w215 -> [w237]
          tunnel: w217 -> [w228]
          tunnel: w216 -> [w233]
          tunnel: w215 -> [w232]
          tunnel: w214 -> [w231]
          tunnel: w213 -> [w230]
          tunnel: w212 -> [w229]
          tunnel: w210 -> [w227]
          shift-right: [w225] -> _
          shift-left: w206 -> [w226]
          tunnel: w204 -> [w224]
          tunnel: w203 -> [w223]
          stop <- w234 stop-if-true
          n248 = case shown="\"Drift Correction\"" w237 {
            selector: w237 -> [_ _ _ w278 w306 _ _ _ _ _ _ _ _ _ _]
            tunnel: [4Pi_Capture_Actions."Quit" ("y") 4Pi_Capture_Actions."Open Shutters" ("y") 4Pi_Capture_Actions."Close Shutters" ("y") w269 w300 4Pi_Capture_Actions."Start Acquisition" ("y") w366 4Pi_Capture_Actions."Setup" ("y") 4Pi_Capture_Actions."Camera" ("y") w432 w465 4Pi_Capture_Actions."Setup" ("y") w520 4Pi_Capture_Actions."Setup" ("y") 4Pi_Capture_Actions."Quit" ("y")] -> w236
            tunnel: [w239 w242 w259 w280 w304 w327 w368 w398 w423 w441 w492 w508 w533 w553 TRUE] -> w234
            tunnel: FALSE -> [w239 w242 w259 w280 w304 w327 w368 w398 w423 w441 w492 w508 w533 w553 _]
            tunnel: w233 -> [_ _ w252 _ _ w312 w367 _ _ w429 _ _ _ _ _]
            tunnel: w232 -> [_ _ w251 _ _ w320 w364 w395 _ _ _ _ _ _ _]
            tunnel: w231 -> [_ _ _ _ w303 _ _ _ _ _ _ _ _ _ _]
            tunnel: w230 -> [_ _ _ w279 _ _ _ _ _ _ _ _ _ _ _]
            tunnel: w229 -> [_ _ _ w274 _ _ _ _ _ _ _ _ _ _ _]
            tunnel: w228 -> [_ _ w249 _ _ w325 w365 w397 _ w433 w472 w506 w531 _ _]
            tunnel: w227 -> [_ _ w245 _ _ _ w363 _ _ _ _ w503 w532 _ _]
            tunnel: w226 -> [w238 w241 w258 w267 w298 w315 w362 w396 w421 w427 w470 w509 w528 w545 w577]
            tunnel: [w238 w241 w258 w267 w298 w315 w361 w396 w421 w427 w491 w509 w528 w545 w577] -> w225
            tunnel: w224 -> [_ _ _ _ _ w308 _ _ _ _ _ _ _ _ _]
            tunnel: w223 -> [_ _ _ _ _ w307 _ _ _ _ _ _ _ _ _]
            frame "Idle", Default {
            }
            frame "Live Preview", "Capture" {
            }
            frame "Abort" {
              w244 = u16 1 ("Current Cycle")
              w253 = FALSE ("Live Preview")
              n249 = call "Orca Flash Messanger.vi"("Notifier Name"=w252, "Camera Actions"=Orca_Flash_Actions."IDLE") -> ()  [unwired: 9 in, 5 out]
              n250 = Equal?(x=4Pi_Capture_Actions."Capture", y=w251) -> (x = y?=w248:bool)
              n251 = Get Notifier Status(notifier=w249) -> (notifier out=w256:refnum<notifier>, current notification=w255:T8)  [unwired: 1 in, 3 out]
              n252 = Bundle By Name(cluster=w255, "Running?"=FALSE) -> (w247:T8)
              n253 = Send Notification(notification=w247, notifier=w256) -> ()  [unwired: 1 in, 2 out]
              n254 = Unbundle By Name(w247) -> ("Init Z Position (µm)"=w246:dbl)
              n255 = case shown="True" w248 {
                tunnel: w246 -> [_ w262]
                tunnel: w245 -> [_ w261]
                frame False {
                }
                frame True {
                  n256 = Build Array(w262) -> (w263:dbl[])
                  n257 = call "Stages Messenger.vi"("Stage Notifier Name"=w261, "Actions"=Stage_Actions."MOVE", "Setpoint"=w263, "Axis"=bool[] [TRUE], "Exit While Busy?"=FALSE) -> ()  [unwired: 7 in, 4 out]
                }
              }
              n258 = local write "Live Preview"(w253) -> ()
              n259 = local write "Capture"(w253) -> ()
              n260 = local write "Current Cycle"(w244) -> ()
              n261 = local write "Current Step"(w244) -> ()
            }
            frame "Open Shutters", "Close Shutters" {
              n262 = Equal?(x=w278, y=4Pi_Capture_Actions."Open Shutters") -> (x = y?=w272:bool)
              n263 = Select(t=Shutter_Actions."Open" ("Action"), s=w272, f=Shutter_Actions."Close") -> (s? t:f=w273:T20)
              n264 = case shown="True" "Auto Shutter" {
                tunnel: w279 -> [_ w287]
                tunnel: w274 -> [_ w282]
                tunnel: w273 -> [_ w281]
                frame False {
                }
                frame True {
                  n265 = flat-sequence {
                    tunnel: w281 -> [w290]
                    tunnel: w287 -> [w291]
                    tunnel: [w291] -> w284
                    tunnel: [w290] -> w283
                    tunnel: w282 -> [w289]
                    tunnel: w281 -> [w288]
                    tunnel: [w294] -> w286
                    tunnel: [w293] -> w285
                    tunnel: w284 -> [w294]
                    tunnel: w283 -> [w293]
                    tunnel: w286 -> [w296]
                    tunnel: w285 -> [w295]
                    frame #0 {
                      n266 = call "Shutter Messenger.vi"("Notifier Name"=w289, "Action"=w288) -> ()  [unwired: 12 in, 2 out]
                    }
                    frame #1 {
                      n267 = Wait (ms)(milliseconds to wait=u32 100) -> ()  [unwired: 1 out]
                    }
                    frame #2 {
                      n268 = call "Shutter Messenger.vi"("Notifier Name"=w296, "Action"=w295) -> ()  [unwired: 12 in, 2 out]
                    }
                  }
                }
              }
              n269 = Select(t=4Pi_Capture_Actions."Laser On" ("y"), s=w272, f=4Pi_Capture_Actions."Laser Off") -> (s? t:f=w269:T9)
            }
            frame "Laser On", "Laser Off" {
              n270 = Equal?(x=w306, y=4Pi_Capture_Actions."Laser On") -> (x = y?=w297:bool)
              n271 = call "AOTF Messenger.vi"("AOTF Notifier Name"=w303, "AOTF Action"=AOTF_Actions."Blank", "Beam Blank"=w297) -> ()  [unwired: 8 in, 5 out]
              n272 = Select(t=4Pi_Capture_Actions."Set Exposure Time" ("y"), s=w297, f=4Pi_Capture_Actions."Quit" ("y")) -> (s? t:f=w300:T9)
            }
            frame "Set Exposure Time" {
              # "Frame Rate (Hz)"
              n273 = Get Notifier Status(notifier=w325) -> (current notification=w321:T8)  [unwired: 1 in, 4 out]
              n274 = Unbundle By Name(w321) -> ("Line Scan?"=w310:bool, "Line Scan Mode"=w309:T3, "Capture Exposure (s)"=w316:dbl, "Preview Exposure (s)"=w317:dbl)
              n275 = Equal?(x=w320, y=4Pi_Capture_Actions."Capture") -> (x = y?=w318:bool)
              n276 = Select(t=w316, s=w318, f=w317) -> (s? t:f=w314:dbl)
              n277 = case shown="True" w310 {
                tunnel: w314 -> [w329 w337]
                tunnel: [w329 w334] -> w313
                tunnel: w312 -> [w328 w336]
                tunnel: [w328 w333] -> w311
                tunnel: w309 -> [_ w332]
                tunnel: w308 -> [_ w331]
                tunnel: w307 -> [_ w330]
                frame False {
                  # "Exposure Time (s)"
                }
                frame True {
                  n278 = To Double Precision Float(number="Number of Lines") -> (double precision float=w335:dbl)
                  n279 = case shown="\"Automatic\"" w332 {
                    tunnel: w337 -> [_ w360]
                    tunnel: w336 -> [w343 w359]
                    tunnel: w335 -> [w341 w358]
                    tunnel: [w339 w357] -> w334
                    tunnel: [w342 w356] -> w333
                    tunnel: w331 -> [_ w349]
                    tunnel: w330 -> [_ w348]
                    frame Default {
                      n280 = call "Orca Flash Messanger.vi"("Notifier Name"=w343, "Camera Actions"=Orca_Flash_Actions."GETPARAM", "sCMOS Parameter"=T15 {"Value"=0.0, "Parameter"=4226016}) -> ("Notifier Name Dup"=w342:string, "sCMOS Parameter"=w346:T15)  [unwired: 8 in, 3 out]
                      n281 = Unbundle By Name(w346) -> ("Value"=w340:dbl)
                      n282 = Multiply(x=w340, y=w341) -> (x*y=w339:dbl)
                    }
                    frame "Automatic" {
                      n283 = call "4Pi Capture Set Interline Interval.vi"("Camera Notifier Name"=w359, "Frame Rate (Hz)"=w360) -> ("Camera Notifier Name (Dup)"=w356:string, "Interline Interval (s)"=w355:dbl)  [unwired: 12 in]
                      n284 = Multiply(x=w355, y=w358) -> (x*y=w357:dbl)
                      n285 = call "4Pi Capture Set Auto Waveform.vi"("Interline Interval"=w355, "Waveform Parameters"=w348) -> ("Offset (V)"=w353:dbl, "Amplitude (V)"=w352:dbl, "Samples per Channel"=w351:i32, "Delay (ms)"=w350:dbl, "Line Scan Settings"=w347:T4)  [unwired: 9 in]
                      n286 = local write "Line Scan Settings"(w347) -> ()
                      n287 = call "AO SCTR Messenger.vi"("Notifier Name"=w349, "Actions"=AO_SCTR_Actions."Update and Run", "Offset (V)"=w353, "Amplitude (V)"=w352, "Samples Per Channel"=w351, "Start Delay (ms)"=w350) -> ()  [unwired: 9 in, 1 out]
                    }
                  }
                }
              }
              n288 = Bundle By Name(cluster=T15 {"Value"=0.0, "Parameter"=2049184} ("sCMOS Parameter"), "Value"=w313) -> (w324:T15)
              n289 = call "Orca Flash Messanger.vi"("Notifier Name"=w311, "Camera Actions"=Orca_Flash_Actions."SETPARAM", "sCMOS Parameter"=w324) -> ()  [unwired: 8 in, 5 out]
            }
            frame "Start Acquisition" {
              n290 = case shown="\"Capture\"" w364 {
                tunnel: w367 -> [_ w371 _]
                tunnel: [4Pi_Capture_Actions."Quit" ("y") 4Pi_Capture_Actions."Quit" ("y") 4Pi_Capture_Actions."Update SubFolder" ("y")] -> w366
                tunnel: w365 -> [_ _ w390]
                tunnel: w363 -> [_ _ w382]
                tunnel: w362 -> [w369 w372 w378]
                tunnel: [w369 w372 w377] -> w361
                frame Default {
                }
                frame "Live Preview" {
                  n291 = call "Orca Flash Messanger.vi"("Notifier Name"=w371, "Camera Actions"=Orca_Flash_Actions."PREVIEW") -> ()  [unwired: 9 in, 5 out]
                }
                frame "Capture" {
                  w376 = sgl 0.0 ("Cycle")
                  n292 = Get Notifier Status(notifier=w390) -> (notifier out=w387:refnum<notifier>, current notification=w388:T8)  [unwired: 1 in, 3 out]
                  n293 = call "Stages Messenger.vi"("Stage Notifier Name"=w382, "Actions"=Stage_Actions."Get Position") -> ("Positions"=w385:dbl[])  [unwired: 10 in, 3 out]
                  n294 = Index Array(array=w385, index=0) -> (element=w383:dbl)
                  n295 = Bundle By Name(cluster=w388, "Init Z Position (µm)"=w383) -> (w379:T8)
                  n296 = Send Notification(notification=w379, notifier=w387) -> ()  [unwired: 1 in, 2 out]
                  n297 = Unbundle By Name(w379) -> ("Cycles"=w380:u16, "No. of Z Steps"=w381:u16)
                  n298 = local write "Z Step"(w376) -> ()
                  n299 = local write "Cycle"(w376) -> ()
                  n300 = local write "Frame"(u32 0 ("Frame")) -> ()
                  n301 = Bundle By Name(cluster=w378, "# of Cycles"=w380, "# of Steps"=w381) -> (w377:T18)
                }
              }
            }
            frame "Update SubFolder" {
              n302 = Equal?(x=w395, y=4Pi_Capture_Actions."Capture") -> (x = y?=w393:bool)
              n303 = And(x=w393, y="Auto Update Subfolder") -> (x .and. y?=w391:bool)
              n304 = case shown="True" w391 {
                tunnel: w397 -> [w404 w420]
                frame False {
                  n305 = Get Notifier Status(notifier=w404) -> (notifier out=w403:refnum<notifier>, current notification=w401:T8)  [unwired: 1 in, 3 out]
                  n306 = Unbundle By Name(w401) -> ("Base Path"=w400:path)
                  n307 = Bundle By Name(cluster=w401, "Save Path"=w400) -> (w402:T8)
                  n308 = Send Notification(notification=w402, notifier=w403) -> ()  [unwired: 1 in, 2 out]
                }
                frame True {
                  n309 = Get Notifier Status(notifier=w420) -> (notifier out=w408:refnum<notifier>, current notification=w407:T8)  [unwired: 1 in, 3 out]
                  n310 = feedback #1(u32 0) -> (w410:u32)
                  n311 = Unbundle By Name(w407) -> ("Base Path"=w419:path)
                  n312 = Increment(x=w410) -> (x+1=w409:u32)
                  n313 = feedback-in #1(w409) -> ()
                  n314 = Format Into String(format string="%03d", w409) -> (resulting string=w411:string)  [unwired: 2 in, 1 out]
                  n315 = Strip Path(path=w419) -> (stripped path=w418:path, name=w416:string)
                  n316 = Concatenate Strings("Subfolder Name", w411) -> (w414:string)
                  n317 = Build Path(base path=w418, name or relative path=w414) -> (appended path=w417:path)
                  n318 = Build Path(base path=w417, name or relative path=w416) -> (appended path=w406:path)
                  n319 = Bundle By Name(cluster=w407, "Save Path"=w406) -> (w405:T8)
                  n320 = Send Notification(notification=w405, notifier=w408) -> ()  [unwired: 1 in, 2 out]
                }
              }
            }
            frame "Setup" {
              # "Change lasers here"
            }
            frame "Camera" {
              n321 = Get Notifier Status(notifier=w433) -> (notifier out=w440:refnum<notifier>, current notification=w425:T8)  [unwired: 1 in, 3 out]
              n322 = property on="Current Laser" class="Ring (strict)"() -> ("RingText.Text"=w424:string)  [unwired: 2 in, 2 out]
              n323 = Unbundle By Name(w427) -> ("Current Cycle"=w431:u16, "Current Step"=w430:u16)
              n324 = Unbundle By Name(w425) -> ("Save Path"=w436:path, "Frames"=w426:u32)
              n325 = call "4Pi Capture File Name Increment.vi"("Step"=w430, "Cycle"=w431, "Laser Line"=w424, "Path In"=w436) -> ("Path Out"=w437:path)  [unwired: 7 in]
              n326 = call "Orca Flash Messanger.vi"("Notifier Name"=w429, "Camera Actions"=Orca_Flash_Actions."Record Settings", "Path"=w437, "# of frames"=w426) -> ("Notifier Name Dup"=w439:string)  [unwired: 7 in, 4 out]
              n327 = call "Orca Flash Messanger.vi"("Notifier Name"=w439, "Camera Actions"=Orca_Flash_Actions."RECORD") -> ("Notifier Name Dup"=w434:string, "Image Ref"=w428:T7)  [unwired: 9 in, 3 out]
              n328 = while {
                tunnel: w434 -> [w462]
                tunnel: [w459] -> w432
                tunnel: w440 -> [w448]
                tunnel: w428 -> [w447]
                stop <- w455 stop-if-true
                n329 = Get Notifier Status(notifier=w448) -> (current notification=w461:T8)  [unwired: 1 in, 4 out]
                n330 = Unbundle By Name(w461) -> ("Running?"=w454:bool)
                n331 = Wait (ms)(milliseconds to wait=u32 25) -> ()  [unwired: 1 out]
                n332 = call "IMAQ Read Custom Data"("Key"="Image Data", "Image"=w447) -> ("Custom Data Out"=w445:string)  [unwired: 7 in, 2 out]
                n333 = Unflatten From JSON(JSON string=w445, type and defaults=T23 {"Frame"=0, "Sensor Height"=0, "Sensor Width"=0, "ROI Height"=0, "ROI Width"=0, "ROI Enable?"=FALSE, "Bit per Pixel"=0} ("Camera IMAQ Key Info")) -> (value=w443:T23)  [unwired: 5 in, 1 out]
                n334 = Not(x=w454) -> (.not. x?=w458:bool)
                n335 = Unbundle By Name(w443) -> ("Frame"=→"Frame" →"Current Frame":u32)
                n336 = Select(t=Orca_Flash_Actions."STATUS" ("Camera Actions"), s=w454, f=Orca_Flash_Actions."IDLE") -> (s? t:f=w449:T17)
                n337 = call "Orca Flash Messanger.vi"("Notifier Name"=w462, "Camera Actions"=w449) -> ("Running?"=w457:bool)  [unwired: 9 in, 4 out]
                n338 = Not(x=w457) -> (.not. x?=w456:bool)
                n339 = Or(x=w458, y=w456) -> (x .or. y?=w455:bool)
                n340 = Select(t=4Pi_Capture_Actions."Switch" ("y"), s=w454, f=4Pi_Capture_Actions."Abort") -> (s? t:f=w459:T9)
              }
            }
            frame "Switch" {
              n341 = Get Notifier Status(notifier=w472) -> (current notification=w471:T8)  [unwired: 1 in, 4 out]
              n342 = Unbundle By Name(w471) -> ("Cycles"=w467:u16, "No. of Z Steps"=w468:u16)
              n343 = Bundle By Name(cluster=w470, "# of Cycles"=w467, "# of Steps"=w468) -> (w469:T18)
              n344 = Unbundle By Name(w469) -> ("Current Cycle"=w481:u16, "# of Cycles"=w480:u16, "Current Step"=w479:u16, "# of Steps"=w478:u16)
              n345 = Increment(x=w481) -> (x+1=w464:u16)
              n346 = Increment(x=w479) -> (x+1=w463:u16)
              n347 = To Single Precision Float(number=w464) -> (single precision float=w477:sgl)
              n348 = To Single Precision Float(number=w480) -> (single precision float=w476:sgl)
              n349 = To Single Precision Float(number=w463) -> (single precision float=w475:sgl)
              n350 = To Single Precision Float(number=w478) -> (single precision float=w474:sgl)
              n351 = Divide(x=w477, y=w476) -> (x/y=→"Cycle":sgl)
              n352 = Divide(x=w475, y=w474) -> (x/y=→"Z Step":sgl)
              n353 = call "4Pi Capture Scan Counter.vi"("Scan Tracker"=w469) -> ("Scan Tracker Out"=w491:T18, "Move stage?"=w484:bool, "F_MVR/T_MOV"=w488:bool, "Exit?"=w490:bool)  [unwired: 7 in]
              n354 = Select(t=4Pi_Capture_Actions."Cycle" ("y"), s=w488, f=4Pi_Capture_Actions."Step") -> (s? t:f=w485:T9)
              n355 = Select(t=w485, s=w484, f=4Pi_Capture_Actions."Setup") -> (s? t:f=w482:T9)
              n356 = Select(t=4Pi_Capture_Actions."Abort" ("y"), s=w490, f=w482) -> (s? t:f=w465:T9)
              n357 = case shown="\"Cycle\"" w465 {
                tunnel: w464 -> [_ w494 _]
                tunnel: w463 -> [_ _ w496]
                frame Default {
                }
                frame "Cycle" {
                  n358 = Increment(x=w494) -> (x+1=→"Current Cycle":u16)
                }
                frame "Step" {
                  n359 = Increment(x=w496) -> (x+1=→"Current Step":u16)
                }
              }
            }
            frame "Step" {
              n360 = Get Notifier Status(notifier=w506) -> (current notification=w505:T8)  [unwired: 1 in, 4 out]
              n361 = Unbundle By Name(w505) -> ("Z Step Size (µm)"=w502:dbl, "No. of Z Steps"=w499:u16)
              n362 = Less?(x=w499, y=u16 2) -> (x < y?=w498:bool)
              n363 = Equal To 0?(x=w502) -> (x = 0?=w501:bool)
              n364 = Build Array(w502) -> (w504:dbl[])
              n365 = Or(x=w501, y=w498) -> (x .or. y?=w500:bool)
              n366 = case shown="False" w500 {
                tunnel: w504 -> [w511 _]
                tunnel: w503 -> [w510 _]
                frame False {
                  n367 = flat-sequence {
                    tunnel: w511 -> [w516]
                    tunnel: w510 -> [w515]
                    frame #0 {
                      n368 = call "Stages Messenger.vi"("Stage Notifier Name"=w515, "Actions"=Stage_Actions."MVR", "Setpoint"=w516, "Axis"=bool[] [TRUE], "Exit While Busy?"=FALSE) -> ()  [unwired: 7 in, 4 out]
                    }
                    frame #1 {
                      n369 = Wait (ms)(milliseconds to wait=u32 75) -> ()  [unwired: 1 out]
                    }
                  }
                }
                frame True {
                }
              }
            }
            frame "Cycle" {
              n370 = Get Notifier Status(notifier=w531) -> (current notification=w530:T8)  [unwired: 1 in, 4 out]
              n371 = Unbundle By Name(w530) -> ("Init Z Position (µm)"=w529:dbl, "Z Step Size (µm)"=w524:dbl, "No. of Z Steps"=w523:u16)
              n372 = Equal To 0?(x=w524) -> (x = 0?=w527:bool)
              n373 = Less?(x=w523, y=u16 2) -> (x < y?=w526:bool)
              n374 = Or(x=w527, y=w526) -> (x .or. y?=w522:bool)
              n375 = case shown="True" w522 {
                tunnel: w532 -> [w535 _]
                tunnel: w529 -> [w534 _]
                frame False {
                  n376 = flat-sequence {
                    tunnel: w535 -> [w541]
                    tunnel: w534 -> [w537]
                    frame #0 {
                      n377 = Build Array(w537) -> (w536:dbl[])
                      n378 = call "Stages Messenger.vi"("Stage Notifier Name"=w541, "Actions"=Stage_Actions."MOVE", "Setpoint"=w536, "Axis"=bool[] [TRUE], "Exit While Busy?"=FALSE) -> ()  [unwired: 7 in, 4 out]
                    }
                    frame #1 {
                      n379 = Wait (ms)(milliseconds to wait=u32 75) -> ()  [unwired: 1 out]
                    }
                  }
                }
                frame True {
                }
              }
              n380 = Select(t=4Pi_Capture_Actions."Drift Correction" ("y"), s="Drift Correction", f=4Pi_Capture_Actions."Setup" ("y")) -> (s? t:f=w520:T9)
            }
            frame "Drift Correction" {
              n381 = Bundle(FALSE, u16 0) -> (w546:cluster{bool, u16})  [unwired: 1 in]
              n382 = Obtain Notifier(name (unnamed)="WFDC External Sync Notifier", notification data type=w546, create if not found? (T)=FALSE) -> (notifier out=w547:refnum<notifier>, error out=w548:errorcluster)  [unwired: 1 in, 1 out]
              n383 = case shown="No Error" w548 {
                selector: w548 -> [w561 w575]
                tunnel: w547 -> [w564 w576]
                tunnel: w546 -> [w566 _]
                tunnel: w545 -> [w559 _]
                tunnel: [w556 w575] -> w543
                tunnel: [w555 w576] -> w544
                frame No Error {
                  n384 = Unbundle By Name(w559) -> ("Current Cycle"=w558:u16)
                  n385 = Increment(x=w558) -> (x+1=w557:u16)
                  n386 = Bundle(cluster=w566, TRUE, w557) -> (w563:cluster{bool, u16})
                  n387 = Send Notification(notification=w563, notifier=w564, error in (no error)=w561) -> (notifier out=w562:refnum<notifier>, error out=w560:errorcluster)
                  n388 = disable-structure shown="Enabled" {
                    disable-tunnel: w562 -> [w572 w574]
                    disable-tunnel: w560 -> [w569 w573]
                    disable-tunnel: [w568 w573] -> w556
                    disable-tunnel: [w567 w574] -> w555
                    frame Disabled {
                      n389 = Wait on Notification(notifier=w572, ignore previous (F)=TRUE, timeout in ms (-1)=30000, error in (no error)=w569) -> (notifier out=w567:refnum<notifier>, error out=w568:errorcluster)  [unwired: 2 out]
                    }
                    frame Enabled {
                    }
                  }
                }
                frame Error {
                }
              }
              n390 = Release Notifier(notifier=w544, error in (no error)=w543) -> ()  [unwired: 1 in, 3 out]
            }
            frame "Quit" {
            }
          }
        }
      }
      n391 = local write "Quit"(w178) -> ()
    }
    frame Error {
      n392 = Release Notifier(notifier=w903) -> (error out=w902:errorcluster)  [unwired: 2 in, 2 out]
      n393 = for {
        tunnel: w901 -> [w908] mode=indexing
        n394 = call "IMAQ Dispose"("Image"=w908) -> ()  [unwired: 5 in, 1 out]
      }
      n395 = Unbundle By Name(w902) -> ("source"=w905:string)
      n396 = Concatenate Strings("4Pi Capture Manager could not start.", "\r", w905) -> (w904:string)
      n397 = One Button Dialog(message=w904) -> ()  [unwired: 1 in, 1 out]
    }
  }
  n398 = control-ref of="This VI"() -> (w86:refnum<vi>)
  n399 = property class="VI"(reference=w86) -> (reference out=w95:refnum<vi>, "Panel"=w87:refnum<vi>)  [unwired: 1 in, 1 out]
  n400 = property class="Pnl"(reference=w87) -> ("Decos[]"=w85:refnum<vi>[], "Panes[]"=w91:refnum<vi>[])  [unwired: 1 in, 2 out]
  n401 = Array Size(array=w85) -> (size(s)=w83:i32)
  n402 = Decrement(x=w83) -> (x-1=w84:i32)
  n403 = Index Array(array=w91, index=0) -> (element=w90:refnum<vi>)
  n404 = Index Array(array=w85, index=w84) -> (element=w93:refnum<vi>)
  n405 = property class="VI"(reference=w95) -> (reference out=w97:refnum<vi>, "Front Panel.PanelBounds"=w98:T25)  [unwired: 1 in, 1 out]
  n406 = property class="Decor"(reference=w93) -> ("Bounds"=w96:T26)  [unwired: 1 in, 2 out]
  n407 = property class="Pane"(reference=w90, "Origin"=T11 {"Horizontal"=0, "Vertical"=0}, "HorizScrollbarVisibility"=w94, "VertScrollbarVisibility"=w94) -> ()  [unwired: 1 in, 2 out]
  n408 = Unbundle By Name(w96) -> ("Width"=w101:u32, "Height"=w104:u32)
  n409 = control-ref of="Quit"() -> (w88:refnum<vi>)
  n410 = To Word Integer(number=w101) -> (16bit integer=w103:i16)
  n411 = To Word Integer(number=w104) -> ()  [unwired: 1 out]
  n412 = property class="Bool (strict)"(reference=w88) -> ("Height"=w106:u32, "Top"=w107:i32)  [unwired: 1 in, 2 out]
  n413 = Unbundle By Name(w98) -> ("Left"=w100:i16, "Top"=w111:i16)
  n414 = To Word Integer(number=w106) -> (16bit integer=w109:i16)
  n415 = To Word Integer(number=w107) -> (16bit integer=w110:i16)
  n416 = Add(x=w100, y=w103) -> (x+y=w102:i16)
  n417 = Compound Arithmetic op=ADD(w111, w109, w110, i16 12 ("y")) -> (w105:i16)
  n418 = Bundle By Name(cluster=w98, "Right"=w102, "Bottom"=w105) -> (w99:T25)
  n419 = property class="VI"(reference=w97, "Front Panel.PanelBounds"=w99) -> ()  [unwired: 1 in, 2 out]
